vi "VP_RT_multiscan.vi"() -> ()   [LabVIEW 2015]
uses:
  Local or Remote.ctl
  State Enum.ctl
  Command Enum.ctl
  Controller Type.ctl
  Scan type.ctl
  EPICS Command Control.ctl
  <vilib>/Platform/TimedLoop/XDataNode/timing_clust.ctl
  <vilib>/Platform/TimedLoop/XDataNode/nitl_modes.ctl
  <vilib>/Platform/TimedLoop/XDataNode/wakeup.ctl
  Data Write Control.ctl
  <vilib>/FPGAPlugInAG/cRIO-9039/niLvFpga_Open_cRIO-9039.vi
  <vilib>/rvi/interface/common/dynamic/niFpgaDynamicAddResources.vi
  <vilib>/Utility/error.llb/Error Cluster From Error Code.vi
  <vilib>/rvi/errors/niLvFpgaAdjustHostInterfaceError.vi
  <vilib>/rvi/interface/common/niFpgaWaitOnOcc.vi
  <vilib>/FPGAPlugInAG/Dynamic/niLvFpga_Reset_Dynamic.vi
  <vilib>/FPGAPlugInAG/Dynamic/niLvFpga_Abort_Dynamic.vi
  <vilib>/FPGAPlugInAG/Dynamic/niLvFpga_Close_Dynamic.vi
  <vilib>/Platform/TimedLoop/XDataNode/XDataNode.xnode
  <vilib>/rvi/interface/nirviOpenFPGA/nirviOpenFPGA.xnode
  FPGA Bitfiles/VP_NanoPositioner_FPGA_Diagonal.lvbitx
  <vilib>/rvi/interface/nirviReadWriteControl/nirviReadWriteControl.xnode
  <vilib>/rvi/interface/nirviMethod/nirviMethod.xnode
  <vilib>/rvi/interface/nirviCloseFPGA/nirviCloseFPGA.xnode
  <vilib>/Platform/TimedLoop/XDataNode/XDNodeRunTimeDep.lvlib
  <vilib>/rvi/errors/niLvFpgaMergeErrorWithErrorCode.vi
  NiFpgaLv.dll
  <vilib>/rvi/interface/Simulation/niFpgaSimulationCallBeginRW.vi
  <vilib>/rvi/Analysis/host/Public/NI_FpgaMspHost.lvlib
  <vilib>/FPGAPlugInAG/Dynamic/niLvFpga_StopFifo_Dynamic.vi
  <vilib>/FPGAPlugInAG/Dynamic/niLvFpga_ReadFifo_Dynamic.vi
  <vilib>/NI_Real-Time Target Support.lvlib
  <vilib>/FPGAPlugInAG/Dynamic/niLvFpga_ConfigureFifo_Dynamic.vi
panel:
  in  "Tab Control":T1(tab)
  in  "Scan type":T2
  in  "Controller Type":T3
  out "Fly Scan Complete":bool
  out "XY actual":cluster{"Array":dbl[], "Array":dbl[]}(graph)
  out "XY Ref":cluster{"Array":dbl[], "Array":dbl[]}(graph)
  out "Elements Available in FIFO":u32(graph)
  out "Elements Remaining in FIFO":u32(graph)
  out "Reference and Actual positions":cluster{"t0":dbl, dbl, dbl[][]}(graph)
  in  "Timeout FPGA FIFO1":i32=40000000
  out "FIFO Timed Out":bool
  out "stop case":bool
  in  "Datalog Cases":T4(ring)=enum."Data Log 16"
  out "FIFO Timed Out?":bool
  out "Number of Elements":u32=1250
  out "Data Read Rate (Hz)":dbl=25000.000000000004
  out "Elements Remaining":u32
  in  "FIFO Timeout (ms)":i32=10000
  out "Actual Depth":u32=131068416
  in  "Requested Depth":u32=131068000
  out "2iddVELO:VP:X_End_nm":dbl=2000.0
  out "2iddVELO:VP:X_Start_nm":dbl=-2000.0
  out "EPICS Execute Command":bool
  out "2iddVELO:VP:Y_Start_nm":dbl=2000.0
  out "2iddVELO:VP:Y_End_nm":dbl=-2000.0
  out "2iddVELO:VP:Y_Step_Size_nm":dbl=50.0
  out "2iddVELO:VP:X_Step_Size_nm":dbl=50.0
  out "2iddVELO:VP:Trigger_Freq_Hz":dbl=1000.0
  out "2iddVELO:VP:Trig_DutyCycle_Per":dbl=99.0
  out "Iteration Duration RT Timed-Loop":i64=128
  in  "X Ramp Start (nm)":fxp<+/-,16,16>=-500.0
  in  "X Ramp End (nm)":fxp<+/-,16,16>=500.0
  in  "X Start Marker (nm)":fxp<+/-,58,25>
  in  "Y Ramp Start (nm)":fxp<+/-,16,16>=500.0
  in  "Y Ramp End (nm)":fxp<+/-,16,16>=-500.0
  in  "Y Step Size (nm)":fxp<+/-,16,16>=50.0
  in  "Y Start Marker (nm)":fxp<+/-,58,25>
  out "Fly Scan Running":bool
  out "Continue Run":bool
  out "X Ramp Period (usec)":fxp<+,24,24>=60000.0
  out "Y Ramp Period (usec)":fxp<+,24,24>=60000.0
  out "# of Hor Lines":fxp<+/-,34,18>=181.0 format="%.22g"
  in  "X Step Size (nm)":fxp<+/-,16,16>=50.0
  out "# of Points per Line":fxp<+/-,33,17>=180.0
  out "# Total Trigger Points":fxp<+/-,64,34>=32580.0
  out "sec per line":dbl=0.06
  out "line per sec (Hz)":dbl=16.666666666666668
  out "X Ramp Period DBL (usec)":dbl=60000.0 format="%#_6f"
  out "Total Scan Time (sec)":dbl=10.86
  in  "Controller Time Period (uSec)":u32=40
  in  "Controller Output Time Period (uSec)":u32=40
  in  "X Reference Time Period (uSec)":u32=40
  in  "Plant Output Time Period (uSec)":u32=40
  in  "Stop System (Careful!!)":bool
  in  "Datalog Time Period (uSec)":u32=40
  in  "Analog Input Time Period (uSec)":u32=40
  in  "Detector Trigger Time Period (uSec)":u32=40
  in  "Trigger Generation Time Period (uSec)":u32=40
  in  "Y Reference Time Period (uSec)":u32=40
  in  "Z Reference Time Period (uSec)":u32=40
  in  "Data Trigger Time Period (uSec)":u32=40
  in  "Reset All":bool
  in  "System Loop Type":enum16{"Open Loop", "Closed Loop"}(ring)
  in  "Base name":string="base_name"
  out "Trigger for Data":fxp<+/-,58,25>=1.0
  out "Data":fxp<+/-,58,25>[](array[numeric])
  out "Number of Data Strings":i32=5
  out "Mod6/DIO3":bool
  out "Mod5/DIO3":bool
  out "Mod4/DIO3":bool
  in  "Sample Z Stage Resolution (nm)":fxp<+,33,3>=0.5
  in  "Sample Y Stage Resolution (nm)":fxp<+,33,3>=0.5
  in  "Sample X Stage Resolution (nm)":fxp<+,33,3>=0.5
  in  "Optics Z Stage Resolution (nm)":fxp<+,33,3>=0.5
  in  "Optics Y Stage Resolution (nm)":fxp<+,33,3>=0.5
  in  "Optics X Stage Resolution (nm)":fxp<+,33,3>=0.5
  in  "Sample Z Reset":bool
  in  "Sample Y Reset":bool
  in  "Sample X Reset":bool
  out "Mod6/DIO2":bool
  out "Mod6/DIO1":bool
  out "Mod6/DIO0":bool=TRUE
  out "Mod5/DIO2":bool
  out "Mod5/DIO1":bool=TRUE
  out "Mod5/DIO0":bool
  out "Mod4/DIO2":bool=TRUE
  out "Mod4/DIO1":bool
  out "Mod4/DIO0":bool=TRUE
  in  "Optics Z Reset":bool
  in  "Optics Y Reset":bool
  in  "Optics X Reset":bool
  in  "Detector Trigger Lower Limit (V)":fxp<+/-,20,5>
  in  "Detector Trigger Upper Limit (V)":fxp<+/-,20,5>=5.0
  out "Detector Trigger (V)":fxp<+/-,20,5>
  out "Detector Trigger In Range?":bool=TRUE
  in  "Trigger High Period (usec)":fxp<+/-,64,45>=1250.0
  in  "Trigger Low Period (usec)":fxp<+/-,64,45>=1250.0
  in  "Trigger High Level (V)":fxp<+/-,20,5>=5.0
  in  "Trigger Low Level (V)":fxp<+/-,20,5>
  in  "Trigger Wave Generator":T5(ring)=enum."Square Wave 1"
  in  "DT Reference Amplitude (V)":fxp<+/-,40,17>=5.0
  in  "DT Reference DC Offset (V)":fxp<+/-,16,16>
  out "DT Frequency (periods/tick)":fxp<+,32,0>=7.500010542571545e-05
  out "DT Phase Offset (periods)":fxp<+,32,0>
  in  "DT Reset":bool
  out "DT Duty Cycle (periods)":fxp<+,32,0>=0.8799999998882413
  in  "DT phase offset (deg)":dbl format="%#.6g"
  in  "DT Frequency (Hz)":dbl=200.0 format="%#_6p"
  in  "DT duty cycle (%)":dbl=88.0 min=0.0 max=100.0 step=1.0
  in  "Z White Noise Seed":u32=4
  in  "Z White Noise Amplitude":u16=32767
  in  "Y White Noise Seed":u32=4
  in  "Y White Noise Amplitude":u16=32767
  in  "Z Reference Reset":bool
  in  "Y Reference Reset":bool
  in  "X Reference Reset":bool
  in  "Z Reference Wave Selection":T6(ring)=enum."Sine Wave"
  in  "X Reference Wave Selection":T7(ring)=enum."Custom Up Down Ramp"
  in  "Y Reference Wave Selection":T8(ring)=enum."Custom Ramp Wave"
  out "Z phase offset (periods)":fxp<+,32,0>
  out "Z frequency (periods/tick)":fxp<+,32,0>=1.25030055642128e-07 format="%.32g"
  in  "Z phase offset (deg)":dbl format="%#.6g"
  in  "Z frequency (Hz)":dbl=5.0 format="%#_6p"
  out "Y phase offset (periods)":fxp<+,32,0>
  out "Y frequency (periods/tick)":fxp<+,32,0>=5.005858838558197e-08 format="%.32g"
  in  "Y phase offset (deg)":dbl format="%#.6g"
  in  "Y frequency (Hz)":dbl=2.0 format="%#_6p"
  out "Z Stage Reference (nm)":fxp<+/-,58,25>
  out "Y Stage Reference (nm)":fxp<+/-,58,25>
  out "X Stage Reference (nm)":fxp<+/-,58,25>
  in  "X White Noise Seed":u32=4
  in  "X White Noise Amplitude":u16=32767
  in  "Z Reference DC Offset (nm)":fxp<+/-,15,15>
  in  "Y Reference DC Offset (nm)":fxp<+/-,16,16>
  in  "X Reference DC Offset (nm)":fxp<+/-,16,16>
  in  "Z Reference Amplitude (nm)":fxp<+/-,40,17>
  in  "Y Reference Amplitude (nm)":fxp<+/-,40,17>=100.0
  in  "X Reference Amplitude (nm)":fxp<+/-,40,17>=100.0
  out "X phase offset (periods)":fxp<+,32,0>
  out "X frequency (periods/tick)":fxp<+,32,0>=1.25030055642128e-07 format="%.32g"
  in  "X phase offset (deg)":dbl format="%#.6g"
  in  "X frequency (Hz)":dbl=5.0 format="%#_6p"
  in  "Scaling mV to V":fxp<+,33,10>=0.001000046730041504
  out "Heartbeat":bool=TRUE
  in  "System command":T9
  in  "Execute":bool
  out "Last Command Executed":T9
  in  "Optics and or Sample Stage":T10(ring)
  out "Remote Mode":bool
  in  "Local_Lock":bool
  out "Local or EPICS":T11
  out "Output filename":string
  out "Output path":path
  out "FPGA state":T12(ring)
  in  "cRIO data dir":string="/home/lvuser/natinst/data"
  out "RT Main Loop State":T13
  out "cRIO path":path
  out "Trigger Frequency (Hz)":dbl
  out "Trigger Duty Cycle (%)":dbl
  out "EPICS Scan Type":T2
  out "EPICS Controller Type":T3
  out "EPICS cRIO Command":T14
  out "Scan loop dt":i64
  in  "FIFO Timeout ratio":dbl=0.05
  in  "Z-Stage Scaling Direction":fxp<+/-,3,3>=-1.0
  in  "Y-Stage Scaling Direction":fxp<+/-,3,3>=-1.0
  in  "Mod 3 AI2 V to nm Scaling":fxp<+,47,18>=1000.0
  in  "Mod 3 AI1 V to nm Scaling":fxp<+,47,18>=1000.0
  in  "Mod 3 AI0 V to nm Scaling":fxp<+,47,18>=1000.0
  out "PI Z-Stage Input (V)":fxp<+/-,20,5>=-0.000732421875
  out "PI Y-Stage Input (V)":fxp<+/-,20,5>=0.005584716796875
  out "PI X-Stage Input (V)":fxp<+/-,20,5>=-0.00311279296875
  in  "Z-Stage nm to V Scaling":fxp<+/-,32,12>=0.0005397796630859375
  in  "Y-Stage nm to V Scaling":fxp<+/-,32,12>=0.0014200210571289062
  in  "X-Stage Scaling Direction":fxp<+/-,3,3>=-1.0
  in  "X-Stage nm to V Scaling":fxp<+/-,32,12>=0.0005359649658203125
  in  "Controller Output Lower Limit":fxp<+/-,20,5>=-5.0
  in  "Controller Output Upper Limit":fxp<+/-,20,5>=5.0
  in  "FPGA Wait Timer (ms)":u16=50
  in  "Pre-Scan pause (ms)":u32=250
  in  "Readback Loop time between iterations (ms)":u32=10
  out "Measured Datalog Time Period (Ticks)":u32=1600
  out "Measured Datalog Loop Rate (secs)":dbl=3.9999999999999996e-05
  out "Measured Datalog Loop Rate (kHz)":dbl=25.000000000000004
  out "Measured Counter Loop Rate (secs)":dbl
  out "Measured Counter Loop Rate (MHz)":dbl=inf
  out "Measured X Reference Loop Rate (secs)":dbl=3.9999999999999996e-05
  out "Measured X Reference Loop Rate (kHz)":dbl=25.000000000000004
  out "Measured X Reference Time Period (Ticks)":u32=1600
  out "Measured Controller Loop Rate (kHz)":dbl=25.000000000000004
  out "Measured Controller Output Loop Rate (secs)":dbl=3.9999999999999996e-05
  out "Measured Controller Output Loop Rate (kHz)":dbl=25.000000000000004
  out "Measured Plant Output Loop Rate (secs)":dbl=3.9999999999999996e-05
  out "Measured Plant Output Loop Rate (kHz)":dbl=25.000000000000004
  out "Measured Controller Loop Rate (secs)":dbl=3.9999999999999996e-05
  out "Measured Controller Time Period (Ticks)":u32=1600
  out "Data Read Period (sec)":dbl=3.9999999999999996e-05
  out "Measured Controller Output Time Period (Ticks)":u32=1600
  out "Measured Plant Output Time Period (Ticks)":u32=1600
  out "Measured Counter Time Period (Ticks)":u32
  out "32 bit Count Optics X":i32
  out "32 bit Count Optics  Y":i32
  out "32 bit Count Optics  Z":i32
  out "32 bit Count Sample X":i32
  out "32 bit Count Sample  Y":i32=2
  out "32 bit Count Sample  Z":i32=-4
  out "Optics X Stage Displacement (nm)":fxp<+/-,58,25>=-1.0
  out "Optics Y Stage Displacement (nm)":fxp<+/-,58,25>
  out "Optics Z Stage Displacement (nm)":fxp<+/-,58,25>
  out "Sample X Stage Displacement (nm)":fxp<+/-,58,25>=-0.5
  out "Sample Y Stage Displacement (nm)":fxp<+/-,58,25>=1.5
  out "Sample Z Stage Displacement (nm)":fxp<+/-,58,25>=-1.0
  out "Measured Analog Input Time Period (Ticks)":u32=1600
  out "Measured Analog Input Loop Rate (secs)":dbl=3.9999999999999996e-05
  out "Measured Analog Input Loop Rate (kHz)":dbl=25.000000000000004
  out "Measured Detector Trigger Time Period (Ticks)":u32=1600
  out "Measured Trigger Gen Time Period (Ticks)":u32=1600
  out "Measured Y Reference Time Period (Ticks)":u32=1600
  out "Measured Z Reference Time Period (Ticks)":u32=1600
  out "Measured Y Reference Loop Rate (secs)":dbl=3.9999999999999996e-05
  out "Measured Y Reference Loop Rate (kHz)":dbl=25.000000000000004
  out "Measured Z Reference Loop Rate (secs)":dbl=3.9999999999999996e-05
  out "Measured Z Reference Loop Rate (kHz)":dbl=25.000000000000004
  out "Measured Data Trigger Time Period (Ticks)":u32=1600
  out "X-Stage Input In Range?":bool=TRUE
  out "Y-Stage Input In Range?":bool=TRUE
  out "Z-Stage Input In Range?":bool=TRUE
  in  "file path soscoeff_xx1 Hinf":path=path "/home/lvuser/natinst/controllers/Kxx_1_Gxx_matched_dow_16ord_mVpnm_cd8a3_AvTio9_X5nm_500pm_all_40us_soscof_xx1.mat"
  in  "file path sos gain SF Controller_xx1 Hinf":path=path "/home/lvuser/natinst/controllers/Kxx_1_Gxx_matched_dow_16ord_mVpnm_cd8a3_AvTio9_X5nm_500pm_all_40us_soscof_xx2.mat"
  in  "file path soscoeff_yy1 Hinf":path=path "/home/lvuser/natinst/controllers/Kyy_trial_1_Gyy_matched_dow_8ord_mVpnm_cd8a3_AvTio9_Y5nm_500pm_all_40us_soscof_yy1.mat"
  in  "file path sos gain SF Controller_yy1 Hinf":path=path "/home/lvuser/natinst/controllers/Kyy_trial_1_Gyy_matched_dow_8ord_mVpnm_cd8a3_AvTio9_Y5nm_500pm_all_40us_soscof_yy2.mat"
  in  "file path soscoeff_zz1 Hinf":path=path "/home/lvuser/natinst/controllers/Kzz_1_Gzz_matched_dow_29ord_mVpnm_cd8a3_AvTio9_Z5nm_500pm_all_40us_soscof_zz1.mat"
  in  "file path sos gain SF Controller_zz1 Hinf":path=path "/home/lvuser/natinst/controllers/Kzz_1_Gzz_matched_dow_29ord_mVpnm_cd8a3_AvTio9_Z5nm_500pm_all_40us_soscof_zz2.mat"
  in  "file path soscoeff_xx1 PID":path=path "/home/lvuser/natinst/controllers/Kxx_pid_2_Gxx_tustin_2ord_mVpnm_cd8a3_soscof_xx1.mat"
  in  "file path sos gain SF Controller_xx1 PID":path=path "/home/lvuser/natinst/controllers/Kxx_pid_2_Gxx_tustin_2ord_mVpnm_cd8a3_soscof_xx2.mat"
  in  "file path soscoeff_yy1 PID":path=path "/home/lvuser/natinst/controllers/Kyy_pid_4_Gyy_tustin_2ord_mVpnm_cd8a3_soscof_yy1.mat"
  in  "file path sos gain SF Controller_yy1 PID":path=path "/home/lvuser/natinst/controllers/Kyy_pid_4_Gyy_tustin_2ord_mVpnm_cd8a3_soscof_yy2.mat"
  in  "file path soscoeff_zz1 PID":path=path "/home/lvuser/natinst/controllers/Kzz_pid_2_Gzz_tustin_2ord_mVpnm_cd8a3_soscof_zz1.mat"
  in  "file path sos gain SF Controller_zz1 PID":path=path "/home/lvuser/natinst/controllers/Kzz_pid_2_Gzz_tustin_2ord_mVpnm_cd8a3_soscof_zz2.mat"
  out "-a01(2) xx1c":fxp<+/-,64,9>[](array[numeric])=[0.637785025840232, 0.9924182654286198, 1.8461027816316544, 0.8635404845716299, 1.0670555456779864, 1.6350703383821101, 1.6323955588345012, 1.1102241390539636, 0.0, 0.0, 0.0, 0.0, 0.0, 0.0, 0.0, 0.0, 0.0, 0.0, 0.0, 0.0]
  out "-a02(2) xx1c":fxp<+/-,64,9>[](array[numeric])=[-0.999855815746439, -0.9676991072632725, -0.9642268720534838, -0.9446498323360957, -0.9442808087139987, -0.7547983908829242, -0.6690016013017409, -0.11027986125857198, 0.0, 0.0, 0.0, 0.0, 0.0, 0.0, 0.0, 0.0, 0.0, 0.0, 0.0, 0.0]
  out "b01(2) xx1c":fxp<+/-,64,9>[](array[numeric])=[-0.6378105164532328, -1.0062332697665268, -1.8762916543815855, -0.8616288879491845, -1.0856571140792324, -1.6862585929720944, -1.743591709663851, -0.6129835805090948, 0.0, 0.0, 0.0, 0.0, 0.0, 0.0, 0.0, 0.0, 0.0, 0.0, 0.0, 0.0]
  out "b02(2) xx1c":fxp<+/-,64,9>[](array[numeric])=[0.9999102047610771, 0.9971375605901365, 0.9926840301018772, 0.9509648854364836, 0.9563369558920378, 0.7818900462139817, 0.7642575436257291, 3.0531133177191805e-16, 0.0, 0.0, 0.0, 0.0, 0.0, 0.0, 0.0, 0.0, 0.0, 0.0, 0.0, 0.0]
  out "sos gain SF Controller xx1c":fxp<+/-,42,9>=-0.1625035791657865
  out "-a01(2) yy1c":fxp<+/-,64,9>[](array[numeric])=[1.8740229377643998, 1.3096977339382483, 1.7453886241944765, 0.2668895009727739, 0.0, 0.0, 0.0, 0.0, 0.0, 0.0, 0.0, 0.0, 0.0, 0.0, 0.0, 0.0, 0.0, 0.0, 0.0, 0.0]
  out "-a02(2) yy1c":fxp<+/-,64,9>[](array[numeric])=[-0.9732703278433918, -0.5194903821190732, -0.7453924481836136, -2.7755575615628914e-17, 0.0, 0.0, 0.0, 0.0, 0.0, 0.0, 0.0, 0.0, 0.0, 0.0, 0.0, 0.0, 0.0, 0.0, 0.0, 0.0]
  out "b01(2) yy1c":fxp<+/-,64,9>[](array[numeric])=[-1.8979173162254057, -1.8463149313261074, -1.7151162246453355, -0.006444279582847878, 0.0, 0.0, 0.0, 0.0, 0.0, 0.0, 0.0, 0.0, 0.0, 0.0, 0.0, 0.0, 0.0, 0.0, 0.0, 0.0]
  out "b02(2) yy1c":fxp<+/-,64,9>[](array[numeric])=[0.9969084979865663, 0.9421233904433339, 0.7362048104846675, 0.0, 0.0, 0.0, 0.0, 0.0, 0.0, 0.0, 0.0, 0.0, 0.0, 0.0, 0.0, 0.0, 0.0, 0.0, 0.0, 0.0]
  out "sos gain SF Controller yy1c":fxp<+/-,42,9>=-1.480983349494636
  out "-a01(2) zz1c":fxp<+/-,64,9>[](array[numeric])=[0.6242394224317618, 1.8967038692417004, 0.6659160318030806, 1.7792660019034106, 1.6870099721477447, 0.6417945190222861, 1.4838029149808185, 1.8456549628851837, 1.2189509782386598, 0.9933314517253298, 1.0158915520299678, 0.8863484387433826, 0.026837806879254994, 1.8269783715122585, 0.22448441435364225, 0.0, 0.0, 0.0, 0.0, 0.0]
  out "-a02(2) zz1c":fxp<+/-,64,9>[](array[numeric])=[-0.9983298461163967, -0.9972287452752734, -0.995744457243837, -0.9947210838396919, -0.9925914602095722, -0.9920974045271405, -0.9881915357970101, -0.9800069383591395, -0.9760641145386646, -0.9508624135515895, -0.9242774595356998, -0.655945641403593, -0.008661844724279444, -0.8269827070369743, 0.0, 0.0, 0.0, 0.0, 0.0, 0.0]
  out "b01(2) zz1c":fxp<+/-,64,9>[](array[numeric])=[-0.6245671059510156, -1.897930093390194, -0.6670970070931089, -1.7670265604573054, -1.6833314913922348, -0.6327437892303018, -1.5025901530730128, -1.8636454269915796, -1.1210694827766767, -0.9982206064398196, -1.0326369335418408, -1.1342635673267367, -1.6852506306166828, -0.9843740162364313, -1.7208456881689926e-15, 0.0, 0.0, 0.0, 0.0, 0.0]
  out "b02(2) zz1c":fxp<+/-,64,9>[](array[numeric])=[0.9973135069419645, 0.9951302056171929, 0.9993435624612031, 0.9919371251860779, 0.994931751453586, 0.9881092761723503, 0.9884874399279107, 0.9977145546300196, 0.9725302934743221, 0.9855561672767964, 0.9893454712398023, 0.846212786518208, 0.7855598927779743, 0.0978075435519738, 0.0, 0.0, 0.0, 0.0, 0.0, 0.0]
  out "sos gain SF Controller zz1c":fxp<+/-,42,9>=-0.1988595259608701
  out "error out (Sig Gen)":errorcluster
  out "FPGA error monitor":errorcluster
  out "FPGA end run error":errorcluster
  out "Timed Loop (end error)":errorcluster
  out "error out (Sig Gen) 2":errorcluster
  out "error out (Sig Gen) 3":errorcluster
  out "error out (Sig Gen) 4":errorcluster
  out "Main Loop error":errorcluster
  out "Main Loop Iterations":i32
  out "RT error":errorcluster
  out "Command Loop Error":errorcluster
  out "Readback error":errorcluster
  out "FPGA wait error":errorcluster
  out "Coeff file import error":errorcluster
  out "Readback loop Iterations":i32
  out "Command Loop Iterations":i32
  out "Heartbeat Loop Iterations":i32
  out "EPICS command error":errorcluster
  out "Reduced Array of States":T13[](array[typedef])
  out "2iddVELO:VP:Scan_Type":string
  out "2iddVELO:VP:Controller_Type":string
  out "2iddVELO:VP:cRIO_Command":string
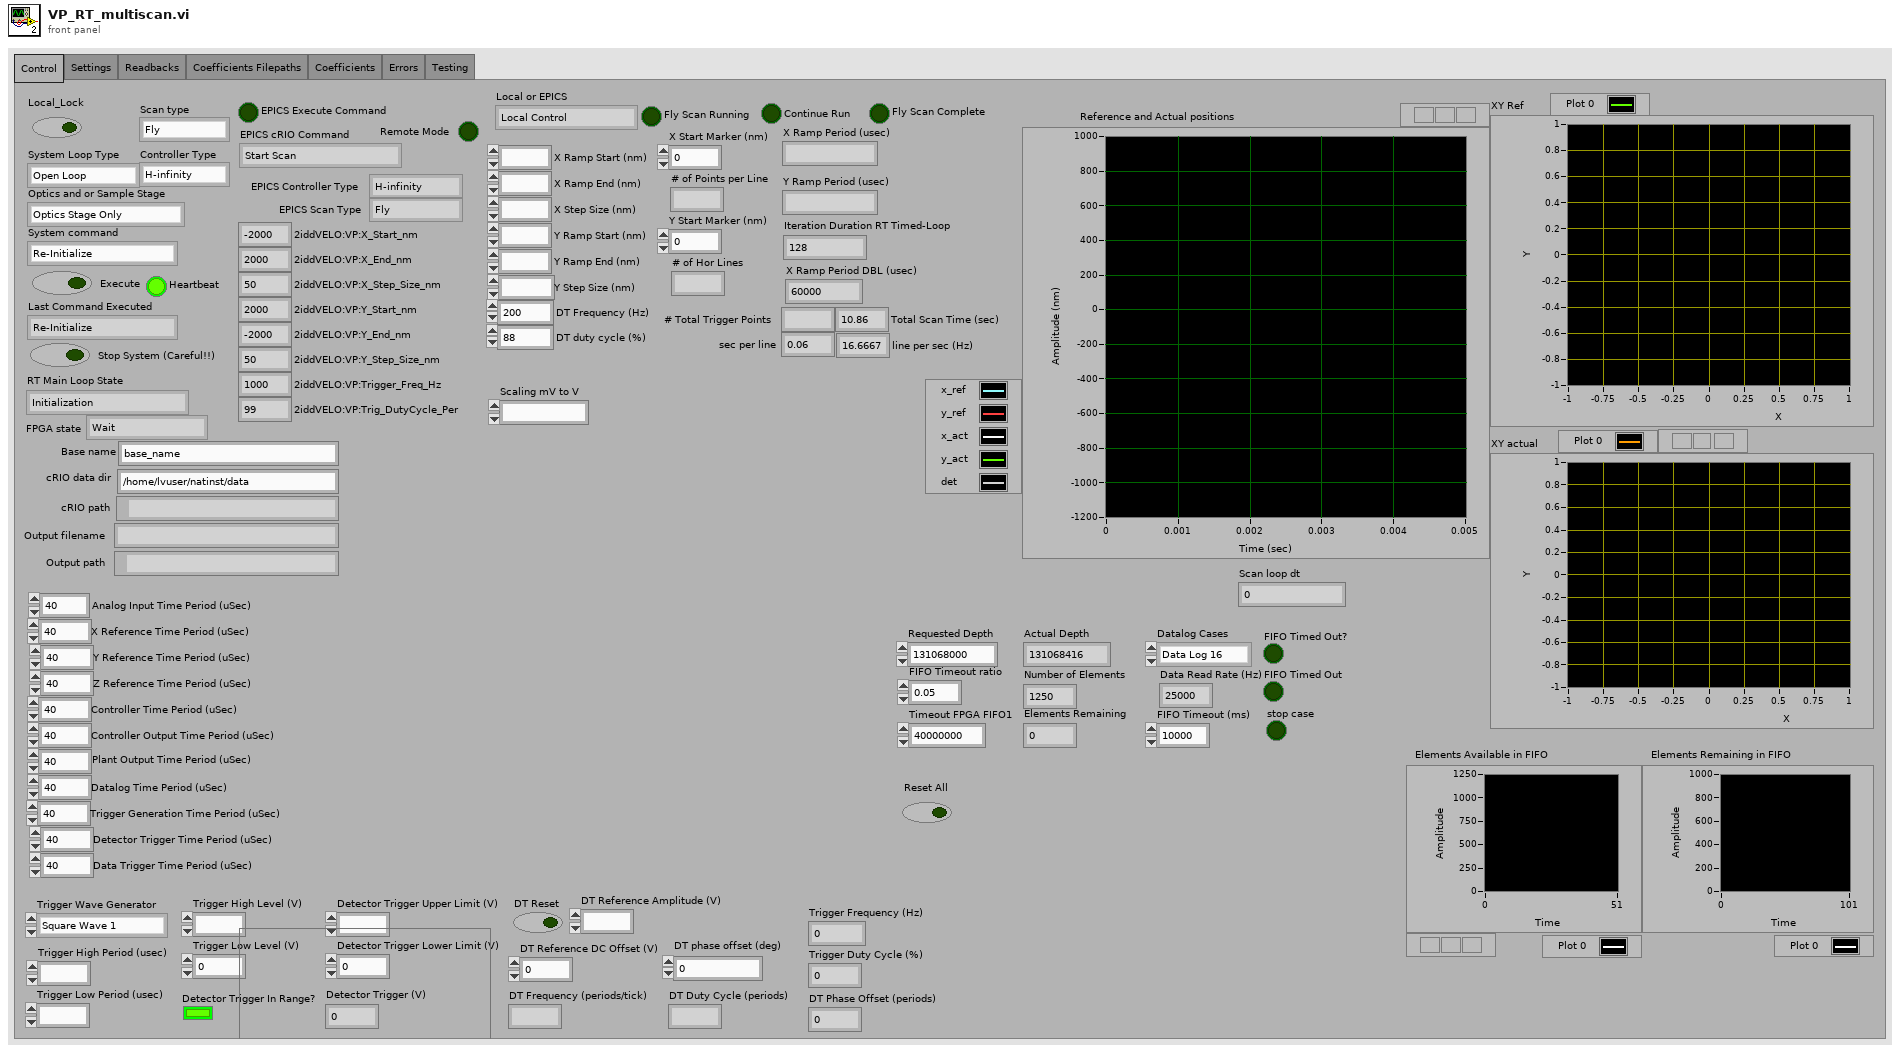
[diagram p1: front panel]
types:
  T1 = enum32{"Control", "Settings", "Readbacks", "Coefficients Filepaths", "Coefficients", "Errors", "Testing"}
  T2 = typedef "Scan type.ctl" = enum16{"Fly", "Step"}
  T3 = typedef "Controller Type.ctl" = enum16{"H-infinity", "PID"}
  T4 = enum16{"Data Log 1", "Data Log 2", "Data Log 3", "Data Log 4", "Data Log 5", "Data Log 6", "Data Log 7", "Data Log 8", "Data Log 9", "Data Log 10", "Data Log 11", "Data Log 12", "Data Log 13", "Data Log 14", "Data Log 15", "Data Log 16"}
  T5 = enum16{"Custom Square Wave ", "Square Wave 1", "Square Wave 2"}
  T6 = enum16{"Constant", "Sine Wave", "Sawtooth Wave", "Square Wave", "Filtered White Noise"}
  T7 = enum16{"Constant", "Sine Wave", "Custom Up Down Ramp", "Filtered White Noise"}
  T8 = enum16{"Constant", "Sine Wave", "Custom Ramp Wave", "Filtered White Noise"}
  T9 = typedef "Command Enum.ctl" = enum16{"Re-Initialize ", "Update Scan Settings", "Scan", "Stop Scan", "Restart FPGA", "Stop System"}
  T10 = enum16{"Optics Stage Only", "Optics and Sample Stage"}
  T11 = typedef "Local or Remote.ctl" = enum16{"Local Control", "EPICS Control"}
  T12 = enum16{"Wait", "Start Run", "Run", "End Run", "Shutdown"}
  T13 = typedef "State Enum.ctl" = enum16{"Initialization", "Import Controller coeffs", "Update Controller Info", "Wait", "Update Reference Info", "Update Detector Trigger Info", "Update Datalog Info", "Check FPGA Status", "Pre-Scan", "Start Scan", "Step Scanning", "Fly Scanning", "End Scan", "Restart FPGA", "Stop FPGA"}
  T14 = typedef "EPICS Command Control.ctl" = enum16{"Start Scan", "Stop Scan", "Reload Controller"}
  T15 = typedef "XDNodeRunTimeDep.lvlib/timing_clust.ctl" = cluster{"Expected End [f-1]":u64, "Actual End [f-1]":u64, "Finished Late? [f-1]":bool, "Expected End [i-1]":u64, "Actual End [i-1]":u64, "Finished Late? [i-1]":bool, "Expected Start [i]":u64, "Actual Start [i]":u64, "Expected Start [f]":u64, "Actual Start [f]":u64, "Source Name":string, "Structure Name":string, "Period":i64, "Deadline":i64, "Offset":i64, "Start":i64, "Priority":i32, "Timeout":i32, "Mode":T16, "Wakeup Reason":T17, "Error":errorcluster, "Source Type":string, "Secondary Source Type":string, "Global End Time":u64, "Global Start Time":u64, "Frame Duration":u64, "Iteration Duration":u64, "Assigned CPU":i32, "I/O Scan Engine Mode":u32}
  T16 = typedef "XDNodeRunTimeDep.lvlib/nitl_modes.ctl" = enum32{"No Change", "Process missed periods, maintain original phase", "Discard missed periods, maintain original phase", "Process missed periods, ignore original phase", "Discard missed periods, ignore original phase"}
  T17 = typedef "XDNodeRunTimeDep.lvlib/wakeup.ctl" = enum32{"Normal", "Aborted", "Asynchronous wakeup", "Timing source error", "Timed loop error", "Timeout"}
  T18 = typedef "Data Write Control.ctl" = enum16{"Initialize", "Read", "Write", "Close"}
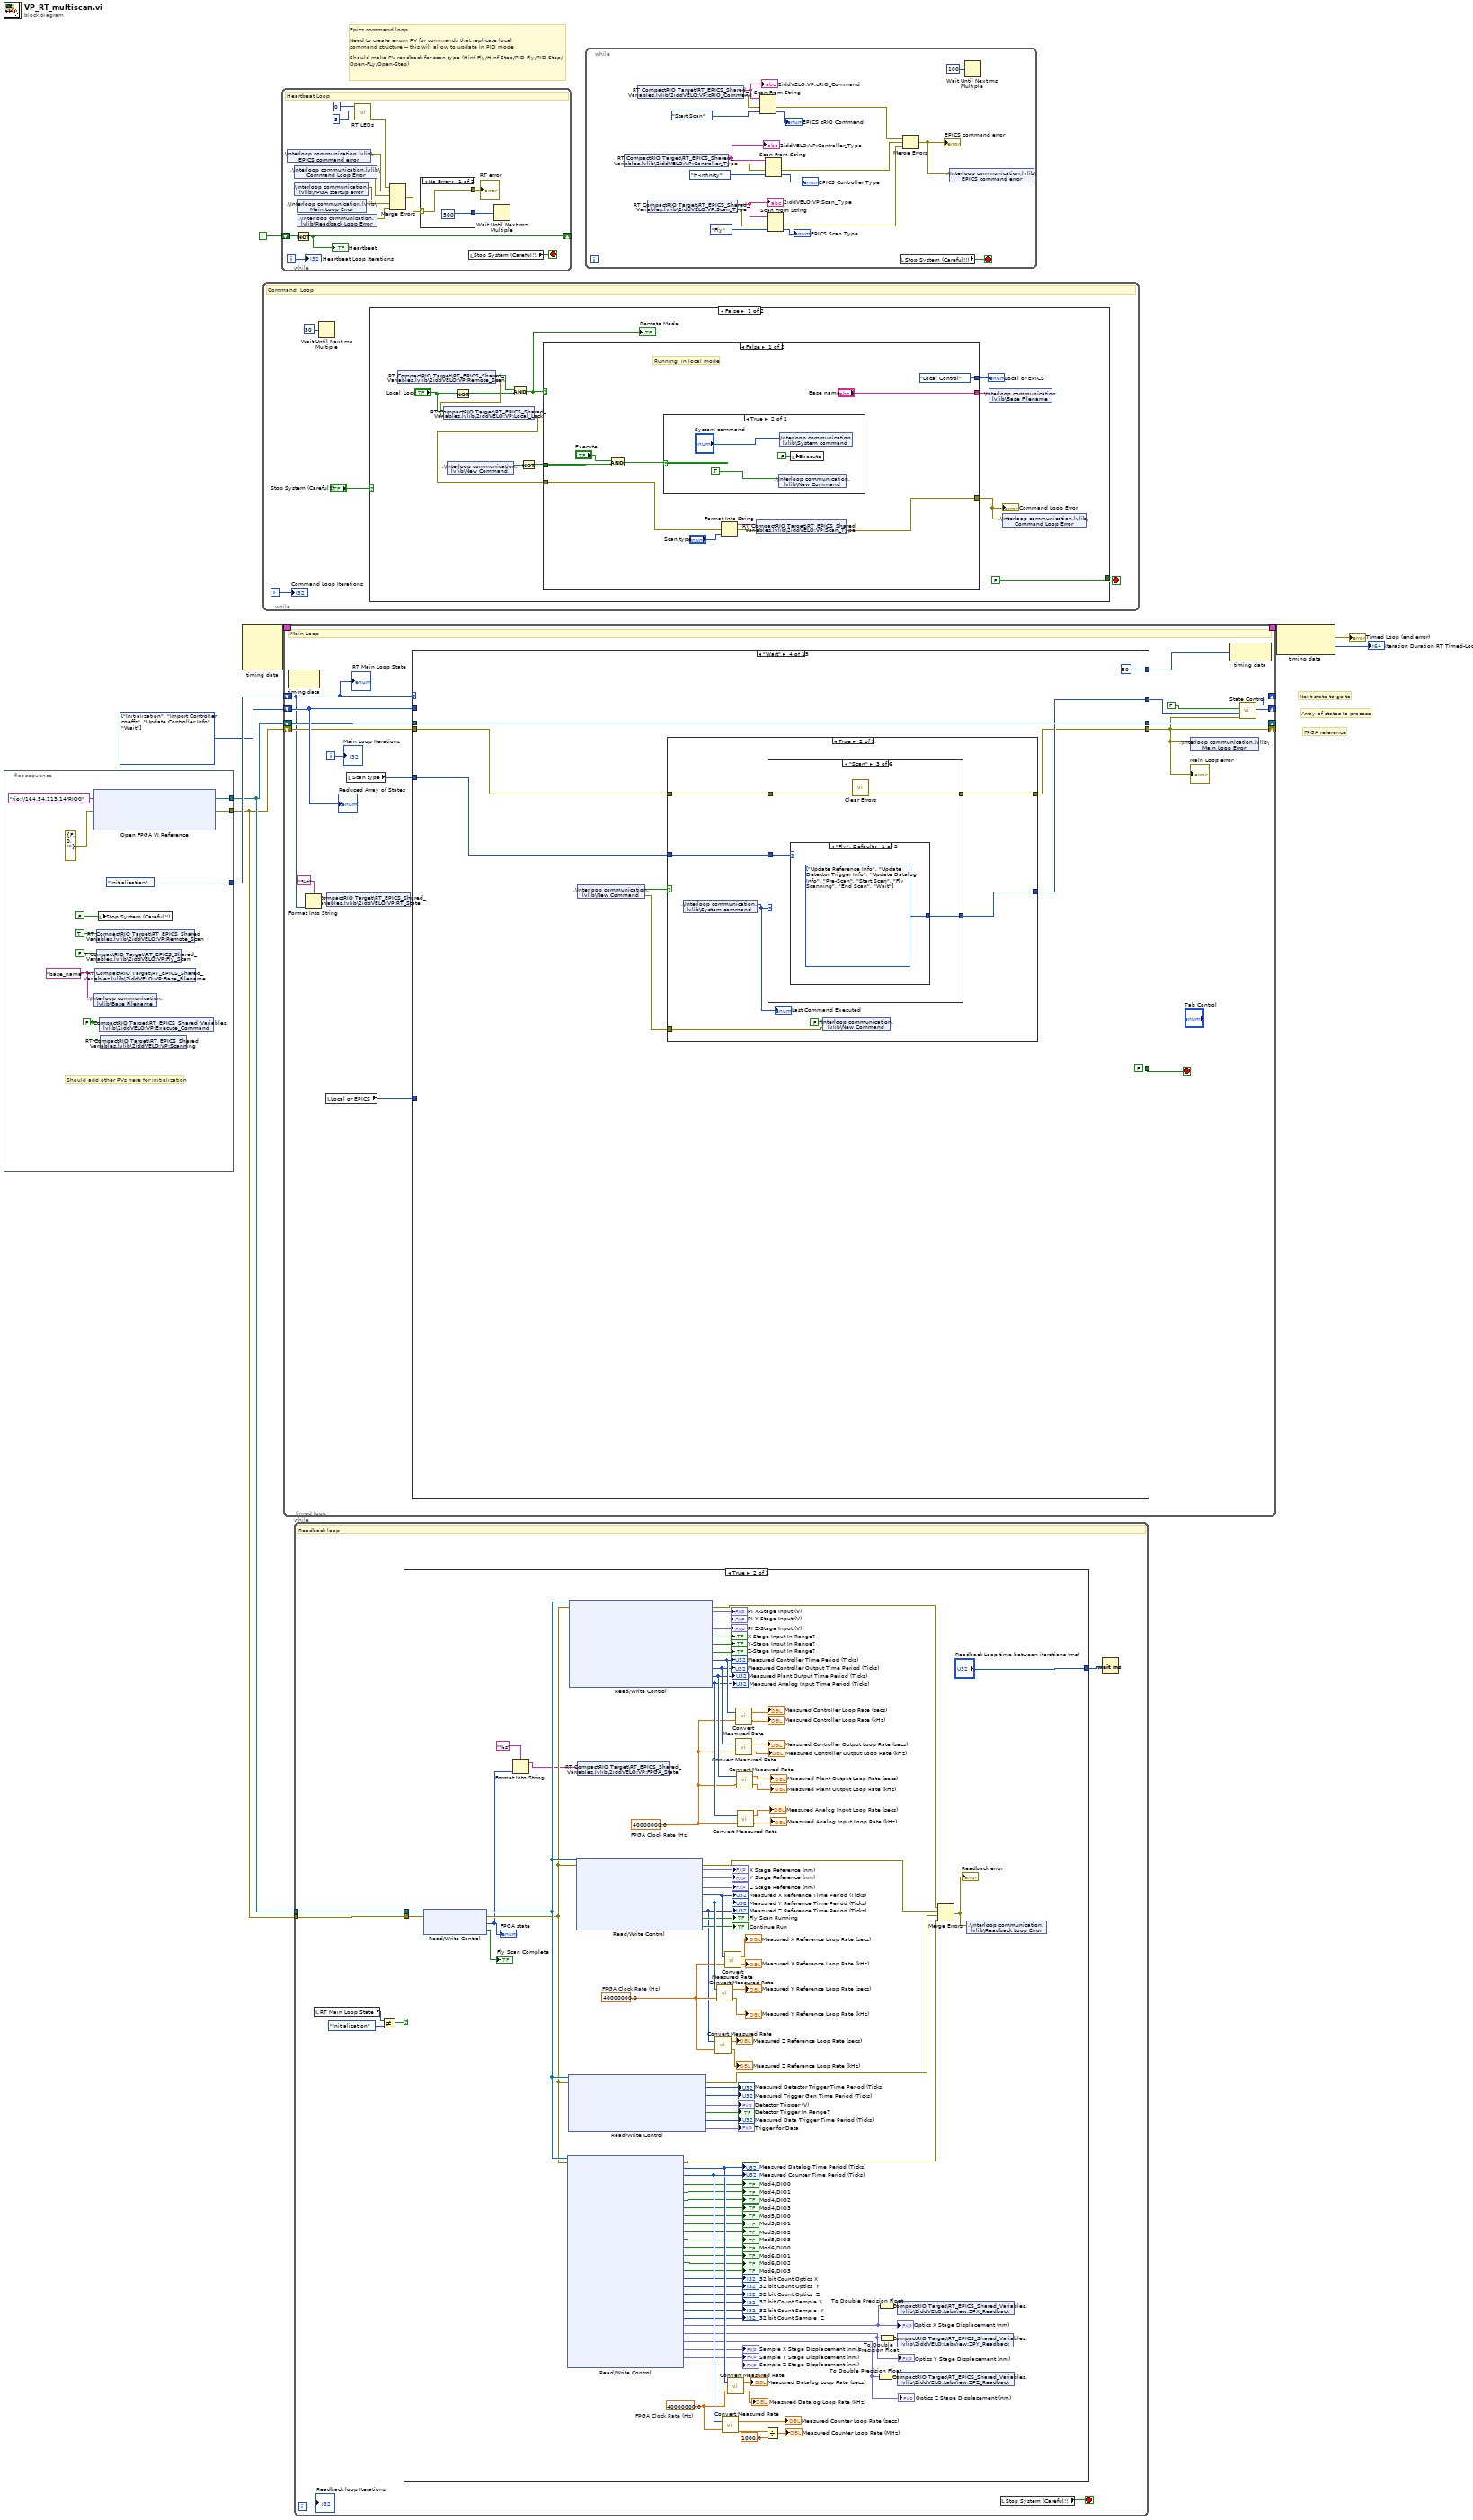
[diagram p0: block diagram]
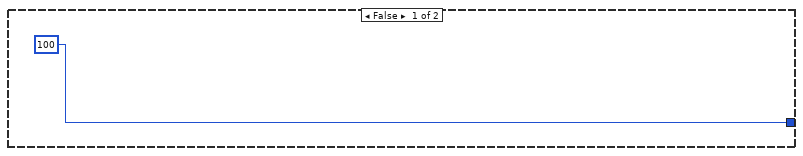
[diagram p2: hidden frame]
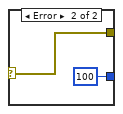
[diagram p3: hidden frame]
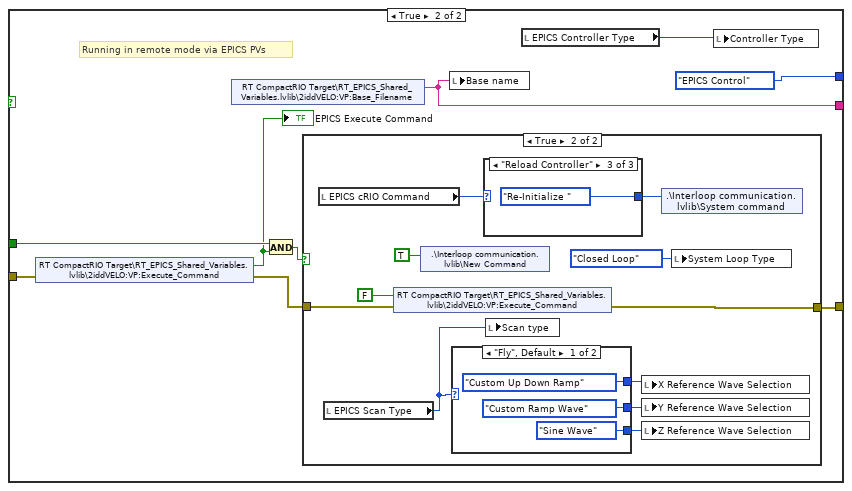
[diagram p5: hidden frame]
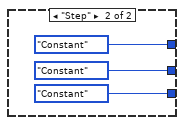
[diagram p7: hidden frame]
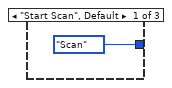
[diagram p8: hidden frame]
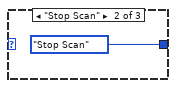
[diagram p9: hidden frame]
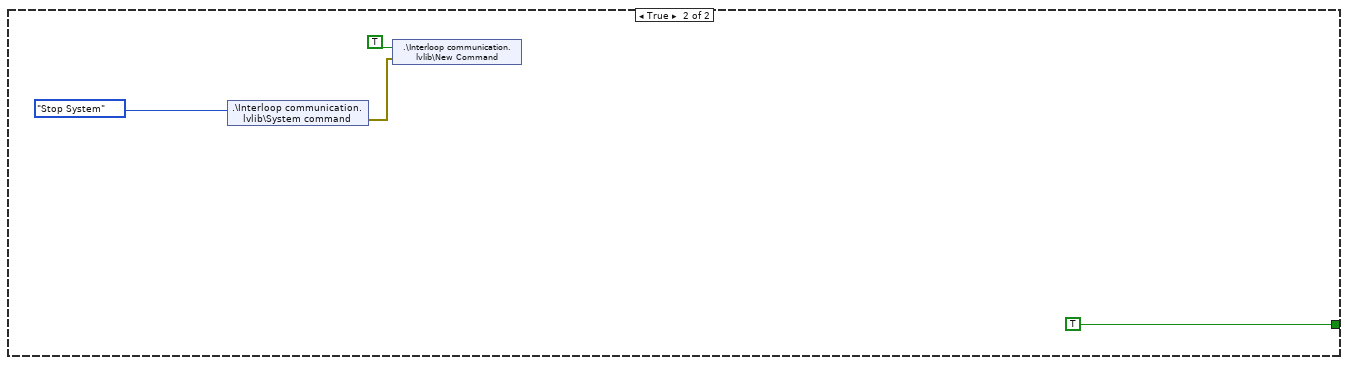
[diagram p10: hidden frame]
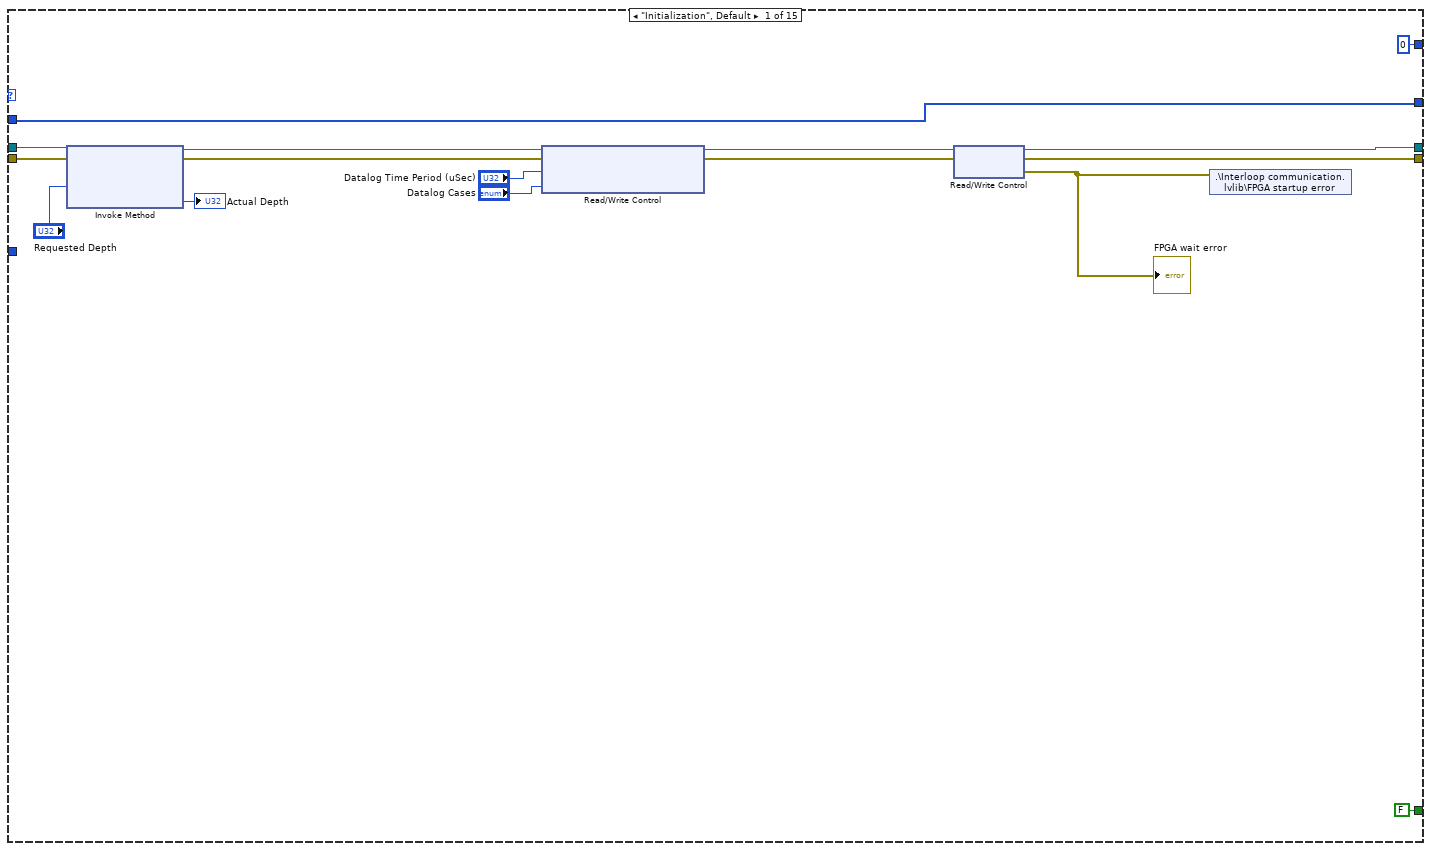
[diagram p11: hidden frame]
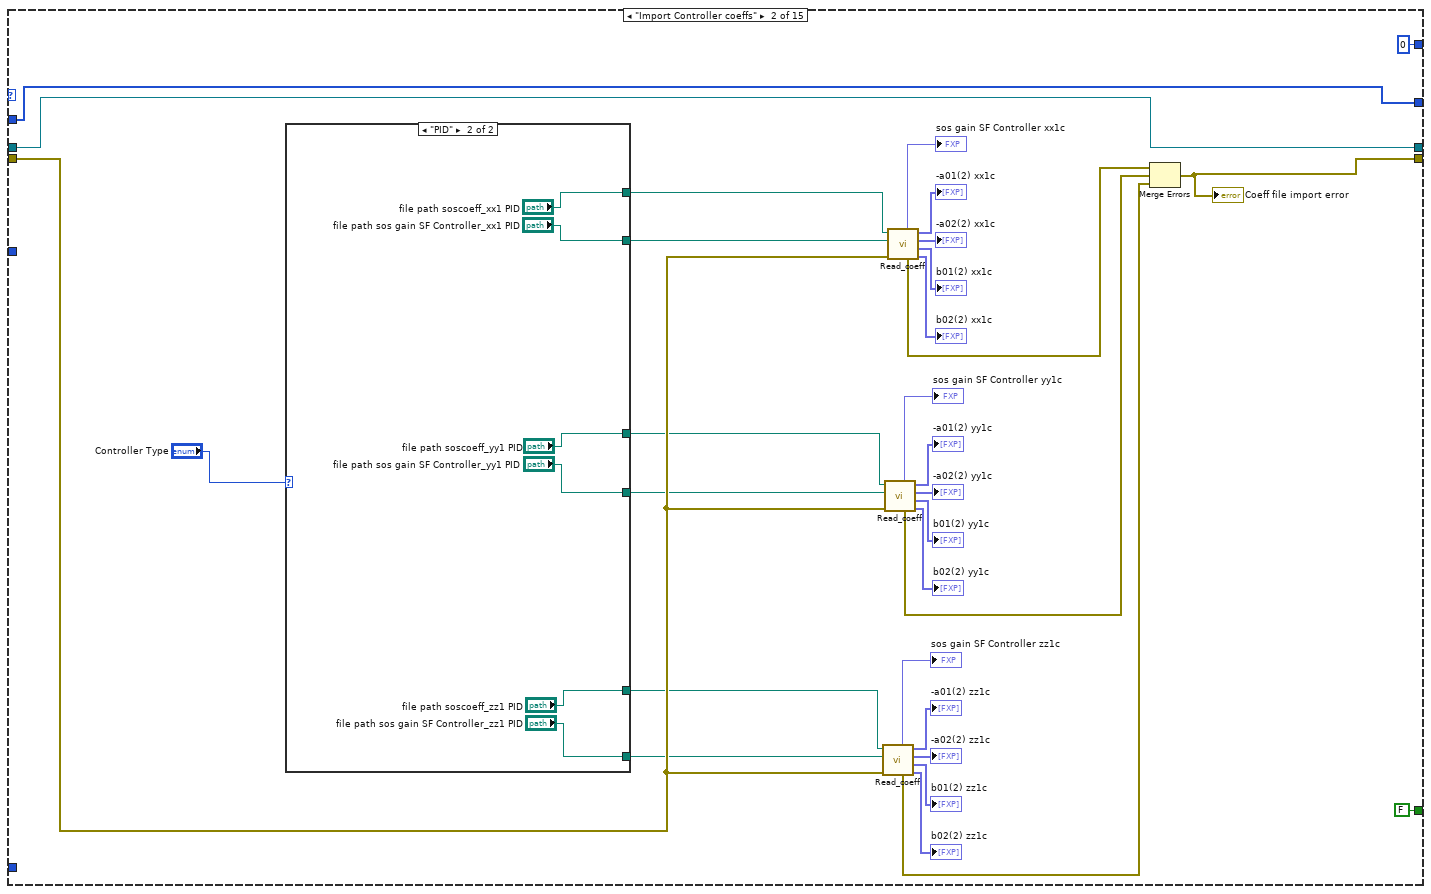
[diagram p12: hidden frame]
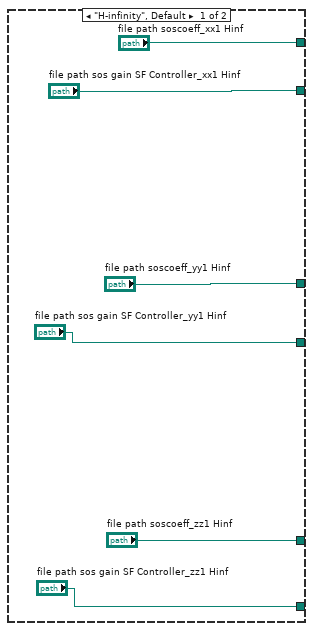
[diagram p13: hidden frame]
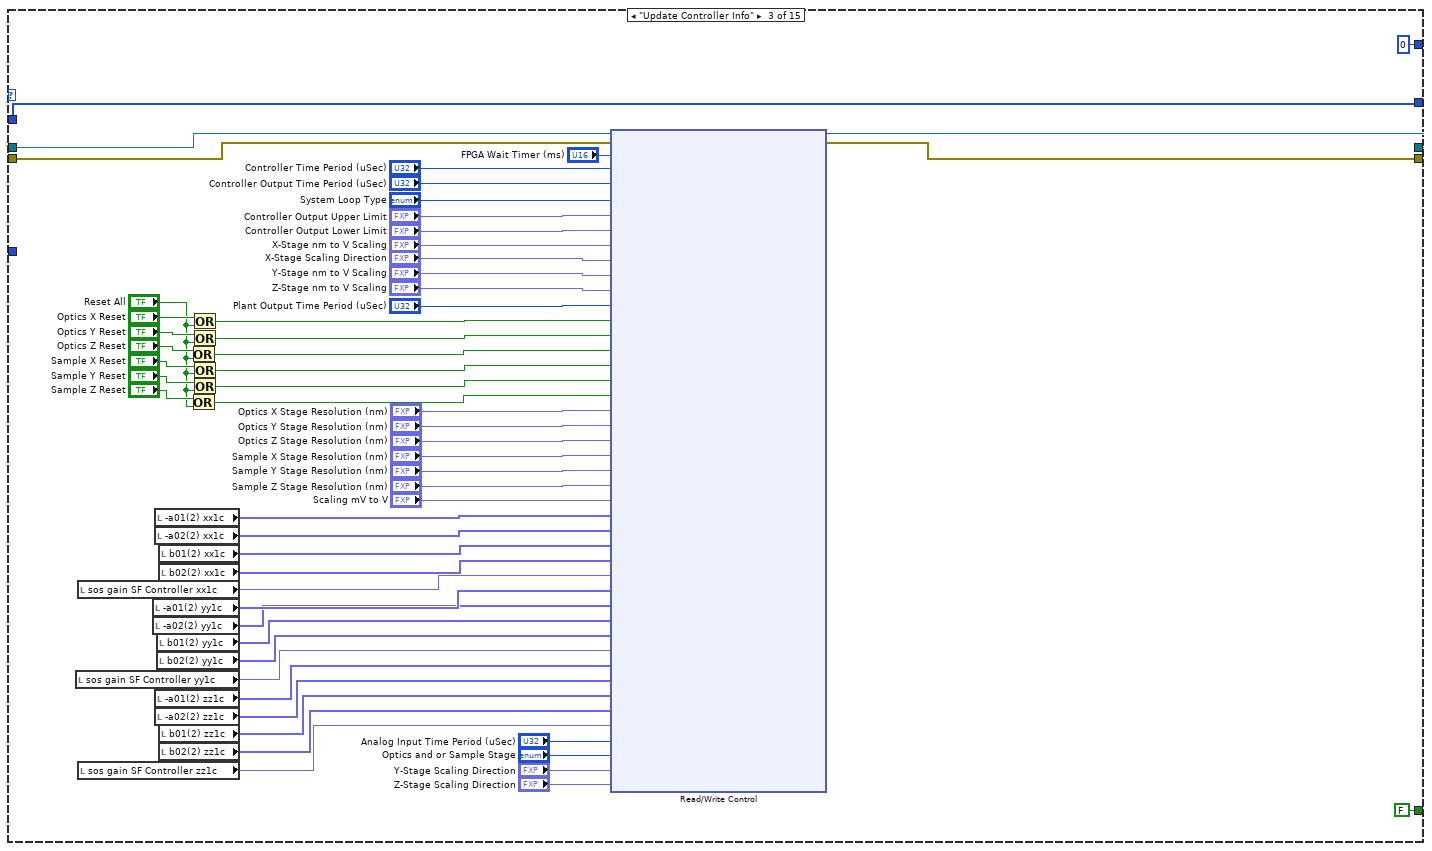
[diagram p14: hidden frame]
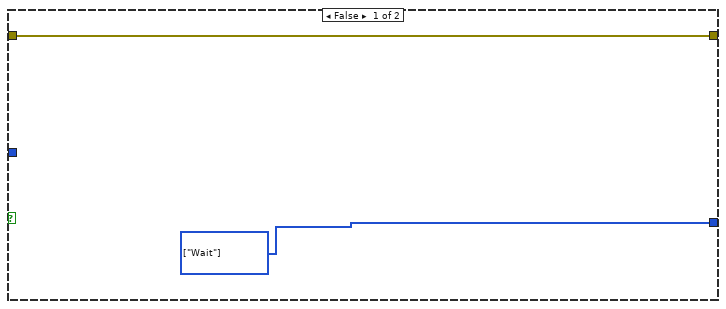
[diagram p15: hidden frame]
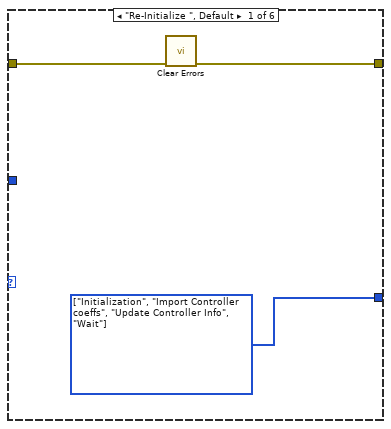
[diagram p16: hidden frame]
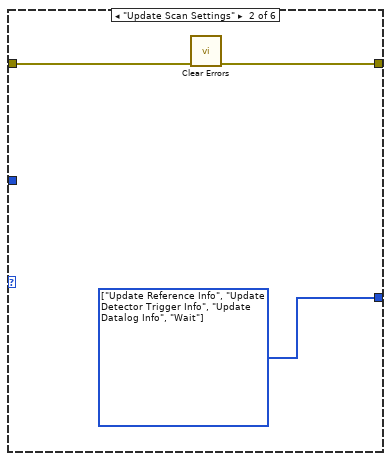
[diagram p17: hidden frame]
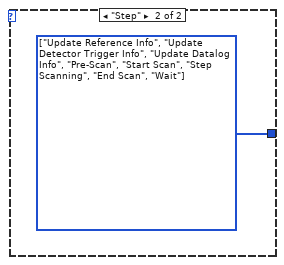
[diagram p18: hidden frame]
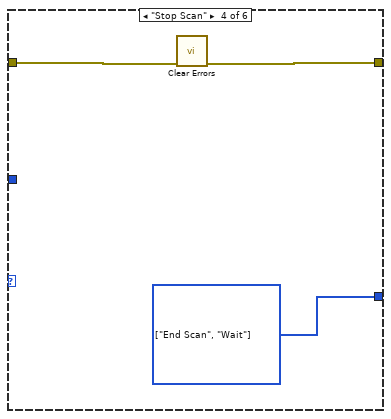
[diagram p19: hidden frame]
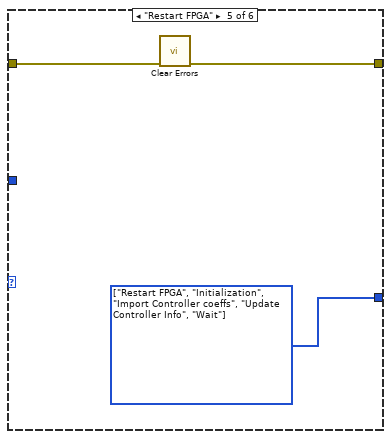
[diagram p20: hidden frame]
diagram:
  w3 = T13[] [enum."Initialization", enum."Import Controller coeffs", enum."Update Controller Info", enum."Wait"] items=["Initialization", "Import Controller coeffs", "Update Controller Info", "Wait", "Update Reference Info", "Update Detector Trigger Info", "Update Datalog Info", "Check FPGA Status", "Pre-Scan", "Start Scan", "Step Scanning", "Fly Scanning", "End Scan", "Restart FPGA", "Stop FPGA"] ("Reduced Array of States")
  # "Epics command loop\n\nNeed to create enum PV for commands that replicate local\ncommand structure -- this will allow to update in PID mode\n\nShould make PV readback for scan type (Hinf-Fly/Hinf-Step/PID-Fly/PID-Step/\nOpen-FLy/Open-Step)"
  # "FPGA reference"
  # "Array of states to process"
  # "Next state to go to"
  n1 = flat-sequence {
    tunnel: [State_Enum."Initialization" ("States")] -> w4
    tunnel: [w16] -> w1
    tunnel: [w15] -> w2
    frame #0 {
      w10 = FALSE ("Start_Scan")
      w13 = "base_name" ("Base_Filename")
      # "Should add other PVs here for initialization"
      n2 = xnode ("Open FPGA VI Reference")("error in"=errorcluster {"status"=FALSE, "code"=0, "source"=""} ("error constant"), "resource name"=tag "rio://164.54.113.14/RIO0") -> ("FPGA VI Reference Out"=w15:refnum<k20>, "error out"=w16:errorcluster)
      n3 = shared-variable ".\\Interloop communication.lvlib\\Base Filename"(w13) -> ()  [unwired: 1 in, 1 out]
      n4 = shared-variable "RT CompactRIO Target\\RT_EPICS_Shared_Variables.lvlib\\2iddVELO:VP:Base_Filename"(w13) -> ()  [unwired: 1 in, 1 out]
      n5 = shared-variable "RT CompactRIO Target\\RT_EPICS_Shared_Variables.lvlib\\2iddVELO:VP:Remote_Scan"(TRUE ("Remote_Scan")) -> ()  [unwired: 1 in, 1 out]
      n6 = shared-variable "RT CompactRIO Target\\RT_EPICS_Shared_Variables.lvlib\\2iddVELO:VP:Fly_Scan"(FALSE ("Fly_Scan")) -> ()  [unwired: 1 in, 1 out]
      n7 = local write "Stop System (Careful!!)"(FALSE ("Stop")) -> ()
      n8 = shared-variable "RT CompactRIO Target\\RT_EPICS_Shared_Variables.lvlib\\2iddVELO:VP:Execute_Command"(w10) -> ()  [unwired: 1 in, 1 out]
      n9 = shared-variable "RT CompactRIO Target\\RT_EPICS_Shared_Variables.lvlib\\2iddVELO:VP:Scanning"(w10) -> ()  [unwired: 1 in, 1 out]
    }
  }
  n10 = node-c288() -> (w9:T15)  [unwired: 4 in]
  n11 = while {
    i -> [w20]
    stop <- w21 stop-if-true
    # "Command  Loop"
    n12 = Wait Until Next ms Multiple(millisecond multiple=u32 50) -> ()  [unwired: 1 out]
    n13 = case shown="False" "Stop System (Careful!!)" {
      tunnel: [FALSE TRUE] -> w21
      frame False {
        n14 = shared-variable "RT CompactRIO Target\\RT_EPICS_Shared_Variables.lvlib\\2iddVELO:VP:Remote_Scan"() -> (w32:bool, error out=w30:errorcluster)  [unwired: 1 in]
        n15 = shared-variable "RT CompactRIO Target\\RT_EPICS_Shared_Variables.lvlib\\2iddVELO:VP:Local_Lock"("Local_Lock", error in=w30) -> (error out=w25:errorcluster)
        n16 = shared-variable ".\\Interloop communication.lvlib\\New Command"() -> (w35:bool)  [unwired: 1 in, 1 out]
        n17 = Not(x="Local_Lock") -> (.not. x?=w27:bool)
        n18 = And(x=w32, y=w27) -> (x .and. y?=w33:bool)
        "Remote Mode" <- w33
        n19 = Not(x=w35) -> (.not. x?=w34:bool)
        n20 = case shown="False" w33 {
          tunnel: w34 -> [w45 w57]
          tunnel: [Local_or_Remote."Local Control" ("Local or EPICS") Local_or_Remote."EPICS Control" ("Local or EPICS")] -> w24
          tunnel: w25 -> [w39 w52]
          tunnel: [w41 w55] -> w29
          tunnel: ["Base name" w54] -> w26
          frame False {
            # "Running  in local mode"
            n21 = And(x="Execute", y=w45) -> (x .and. y?=w43:bool)
            n22 = case shown="True" w43 {
              frame False {
              }
              frame True {
                n23 = shared-variable ".\\Interloop communication.lvlib\\New Command"(TRUE ("New Command")) -> ()  [unwired: 1 in, 1 out]
                n24 = shared-variable ".\\Interloop communication.lvlib\\System command"("System command") -> ()  [unwired: 1 in, 1 out]
                n25 = local write "Execute"(FALSE ("Execute")) -> ()
              }
            }
            n26 = Format Into String(error in=w39, "Scan type") -> (resulting string=w40:string, error out=w38:errorcluster)  [unwired: 2 in]
            n27 = shared-variable "RT CompactRIO Target\\RT_EPICS_Shared_Variables.lvlib\\2iddVELO:VP:Scan_Type"(w40, error in=w38) -> (error out=w41:errorcluster)
          }
          frame True {
            # "Running in remote mode via EPICS PVs"
            n28 = shared-variable "RT CompactRIO Target\\RT_EPICS_Shared_Variables.lvlib\\2iddVELO:VP:Execute_Command"(error in=w52) -> (w53:bool, error out=w51:errorcluster)
            "EPICS Execute Command" <- w53
            n29 = shared-variable "RT CompactRIO Target\\RT_EPICS_Shared_Variables.lvlib\\2iddVELO:VP:Base_Filename"() -> (w54:string)  [unwired: 1 in, 1 out]
            n30 = And(x=w57, y=w53) -> (x .and. y?=w56:bool)
            n31 = case shown="True" w56 {
              tunnel: [w58 w68] -> w55
              tunnel: w51 -> [w58 w65]
              frame False {
              }
              frame True {
                n32 = local read "EPICS cRIO Command"() -> (w66:T14)
                n33 = local read "EPICS Scan Type"() -> (w62:T2)
                n34 = shared-variable "RT CompactRIO Target\\RT_EPICS_Shared_Variables.lvlib\\2iddVELO:VP:Execute_Command"(FALSE ("2iddVELO:VP:Flyscan_Start"), error in=w65) -> (error out=w68:errorcluster)
                n35 = shared-variable ".\\Interloop communication.lvlib\\New Command"(TRUE ("New Command")) -> ()  [unwired: 1 in, 1 out]
                n36 = case shown="\"Fly\", Default" w62 {
                  tunnel: [T7."Custom Up Down Ramp" ("X Reference Wave Selection") T7."Constant" ("X Reference Wave Selection")] -> w61
                  tunnel: [T8."Custom Ramp Wave" ("Y Reference Wave Selection") T8."Constant" ("Y Reference Wave Selection")] -> w60
                  tunnel: [T6."Sine Wave" ("Z Reference Wave Selection") T6."Constant" ("Z Reference Wave Selection")] -> w59
                  frame "Fly", Default {
                  }
                  frame "Step" {
                  }
                }
                n37 = case shown="\"Reload Controller\"" w66 {
                  tunnel: [Command_Enum."Scan" ("System command") Command_Enum."Stop Scan" ("System command") Command_Enum."Re-Initialize " ("System command")] -> w63
                  frame "Start Scan", Default {
                  }
                  frame "Stop Scan" {
                  }
                  frame "Reload Controller" {
                  }
                }
                n38 = local write "Scan type"(w62) -> ()
                n39 = local write "X Reference Wave Selection"(w61) -> ()
                n40 = local write "Y Reference Wave Selection"(w60) -> ()
                n41 = local write "Z Reference Wave Selection"(w59) -> ()
                n42 = shared-variable ".\\Interloop communication.lvlib\\System command"(w63) -> ()  [unwired: 1 in, 1 out]
                n43 = local write "System Loop Type"(enum16{"Open Loop", "Closed Loop"}."Closed Loop" ("System Loop Type")) -> ()
              }
            }
            n44 = local write "Base name"(w54) -> ()
            n45 = local read "EPICS Controller Type"() -> (w50:T3)
            n46 = local write "Controller Type"(w50) -> ()
          }
        }
        "Local or EPICS" <- w24
        "Command Loop Error" <- w29
        n47 = shared-variable ".\\Interloop communication.lvlib\\Base Filename"(w26) -> ()  [unwired: 1 in, 1 out]
        n48 = shared-variable ".\\Interloop communication.lvlib\\Command Loop Error"(w29) -> ()  [unwired: 1 in, 1 out]
      }
      frame True {
        n49 = shared-variable ".\\Interloop communication.lvlib\\System command"(Command_Enum."Stop System" ("System command")) -> (error out=w79:errorcluster)  [unwired: 1 in]
        n50 = shared-variable ".\\Interloop communication.lvlib\\New Command"(TRUE ("New Command"), error in=w79) -> ()  [unwired: 1 out]
      }
    }
    "Command Loop Iterations" <- w20
  }
  n51 = while {
    shift-right: [w96] -> _
    shift-left: TRUE -> [w97]
    i -> [w85]
    stop <- w89 stop-if-true
    # "Heartbeat Loop"
    n52 = shared-variable ".\\Interloop communication.lvlib\\EPICS command error"() -> (w83:errorcluster)  [unwired: 1 in, 1 out]
    n53 = shared-variable ".\\Interloop communication.lvlib\\Command Loop Error"() -> (w91:errorcluster)  [unwired: 1 in, 1 out]
    n54 = shared-variable ".\\Interloop communication.lvlib\\FPGA startup error"() -> (w88:errorcluster)  [unwired: 1 in, 1 out]
    n55 = Not(x=w97) -> (.not. x?=w96:bool)
    "Heartbeat" <- w96
    n56 = shared-variable ".\\Interloop communication.lvlib\\Readback Loop Error"() -> (w90:errorcluster)  [unwired: 1 in, 1 out]
    n57 = shared-variable ".\\Interloop communication.lvlib\\Main Loop Error"() -> (w95:errorcluster)  [unwired: 1 in, 1 out]
    n58 = call <vilib>:"RT LEDs.vi"("State"=3, "LED Num"=0) -> ("error out"=w84:errorcluster)  [unwired: 4 in, 1 out]
    n59 = Merge Errors(w84, w83, w91, w88, w95, w90) -> (w92:errorcluster)
    n60 = case shown="No Error" w92 {
      selector: w92 -> [w98 w100]
      tunnel: [u32 500 ("millisecond multiple") u32 100 ("millisecond multiple")] -> w94
      tunnel: [w98 w100] -> w93
      frame No Error {
      }
      frame Error {
      }
    }
    "RT error" <- w93
    n61 = local read "Stop System (Careful!!)"() -> (w89:bool)
    n62 = Wait Until Next ms Multiple(millisecond multiple=w94) -> ()  [unwired: 1 out]
    "Heartbeat Loop Iterations" <- w85
  }
  n63 = timed-loop {
    timing: w9 -> [_]
    timing-out: [_] -> w8
    shift-right: [w109] -> _
    shift-left: w4 -> [w103]
    shift-right: [w116] -> _
    shift-left: w2 -> [w110]
    shift-right: [w107] -> _
    shift-left: w1 -> [w111]
    shift-right: [w113] -> _
    shift-left: w3 -> [w114]
    i -> [w115]
    stop <- w118 stop-if-true
    # "Main Loop"
    n64 = node-c288() -> ()  [unwired: 1 in, 1 out]
    n65 = Format Into String(format string="%s", w103) -> (resulting string=w104:string)  [unwired: 2 in, 1 out]
    n66 = local read "Local or EPICS"() -> (w108:T11)
    n67 = shared-variable "RT CompactRIO Target\\RT_EPICS_Shared_Variables.lvlib\\2iddVELO:VP:RT_State"(w104) -> ()  [unwired: 1 in, 1 out]
    n68 = local read "Scan type"() -> (w102:T2)
    n69 = case shown="\"Wait\"" w103 {
      tunnel: [w125 w145 w183 w241 w284 w398 w431 w444 w467 w503 w528 w567 w618 w646 w658] -> w117
      tunnel: [FALSE ("Stop") FALSE ("Stop") FALSE ("Stop") FALSE ("Stop") FALSE ("Stop") FALSE ("Stop") FALSE ("Stop") FALSE ("Stop") _ FALSE ("Stop") FALSE ("Stop") FALSE ("Stop") FALSE ("Stop") FALSE ("Stop") TRUE ("Stop")] -> w118
      tunnel: [w128 w150 w182 w243 w282 w397 w430 w446 w458 w495 w521 w588 w605 w641 w655] -> w116
      tunnel: [w120 w147 w181 w237 w281 w396 w429 w437 w457 w498 w520 w586 w617 w640 w660] -> w107
      tunnel: w111 -> [w126 w142 w185 w238 w290 w400 w432 w447 w465 w496 w522 w593 w610 w644 w664]
      tunnel: w110 -> [w127 w150 w184 w243 w291 w401 w433 w448 w466 w494 w523 w589 w612 w650 w665]
      tunnel: w114 -> [w125 w145 w183 _ w284 w398 w431 w444 w467 w503 w529 w568 w618 w646 _]
      tunnel: [i64 0 i64 0 i64 0 i64 50 i64 0 i64 0 i64 0 i64 0 i64 0 i64 250 i64 50 w553 i64 0 i64 0 i64 0] -> w112
      tunnel: w108 -> [_ _ _ _ w278 w393 _ _ _ _ w516 _ _ _ _]
      tunnel: w102 -> [_ _ _ w235 w277 _ _ _ _ w493 _ _ w607 _ _]
      frame "Initialization", Default {
        n70 = xnode "Invoke Method"("FPGA VI Reference In"=w127, "error in"=w126, "Requested Depth"="Requested Depth") -> ("FPGA VI Reference Out"=w130:refnum<k20>, "error out"=w129:errorcluster, "Actual Depth"=→"Actual Depth":u32)
        n71 = xnode "Read/Write Control"("FPGA VI Reference In"=w130, "error in"=w129, "Datalog Time Period (uSec)"="Datalog Time Period (uSec)", "Datalog Cases"="Datalog Cases") -> ("FPGA VI Reference Out"=w122:refnum<k20>, "error out"=w121:errorcluster)
        n72 = xnode "Read/Write Control"("FPGA VI Reference In"=w122, "error in"=w121) -> ("FPGA VI Reference Out"=w128:refnum<k20>, "error out"=w120:errorcluster, "Wait error"=w119:errorcluster)
        "FPGA wait error" <- w119
        n73 = shared-variable ".\\Interloop communication.lvlib\\FPGA startup error"(w119) -> ()  [unwired: 1 in, 1 out]
      }
      frame "Import Controller coeffs" {
        n74 = case shown="\"PID\"" "Controller Type" {
          tunnel: ["file path soscoeff_xx1 Hinf" "file path soscoeff_xx1 PID"] -> w141
          tunnel: ["file path sos gain SF Controller_xx1 Hinf" "file path sos gain SF Controller_xx1 PID"] -> w140
          tunnel: ["file path soscoeff_yy1 Hinf" "file path soscoeff_yy1 PID"] -> w139
          tunnel: ["file path sos gain SF Controller_yy1 Hinf" "file path sos gain SF Controller_yy1 PID"] -> w138
          tunnel: ["file path sos gain SF Controller_zz1 Hinf" "file path sos gain SF Controller_zz1 PID"] -> w137
          tunnel: ["file path soscoeff_zz1 Hinf" "file path soscoeff_zz1 PID"] -> w136
          frame "H-infinity", Default {
          }
          frame "PID" {
          }
        }
        n75 = call "Read_coeff.vi"("error in (no error)"=w142, "sos gain SF controller file path"=w137, "sos coeff file path"=w136) -> ("b02(2)"=→"b02(2) zz1c":fxp<+/-,64,9>[], "b01(2)"=→"b01(2) zz1c":fxp<+/-,64,9>[], "-a02(2)"=→"-a02(2) zz1c":fxp<+/-,64,9>[], "-a01(2)"=→"-a01(2) zz1c":fxp<+/-,64,9>[], "error out"=w146:errorcluster, "sos gain SF Controller"=→"sos gain SF Controller zz1c":fxp<+/-,42,9>)  [unwired: 3 in]
        n76 = call "Read_coeff.vi"("error in (no error)"=w142, "sos gain SF controller file path"=w138, "sos coeff file path"=w139) -> ("b02(2)"=→"b02(2) yy1c":fxp<+/-,64,9>[], "b01(2)"=→"b01(2) yy1c":fxp<+/-,64,9>[], "-a02(2)"=→"-a02(2) yy1c":fxp<+/-,64,9>[], "-a01(2)"=→"-a01(2) yy1c":fxp<+/-,64,9>[], "error out"=w144:errorcluster, "sos gain SF Controller"=→"sos gain SF Controller yy1c":fxp<+/-,42,9>)  [unwired: 3 in]
        n77 = call "Read_coeff.vi"("error in (no error)"=w142, "sos gain SF controller file path"=w140, "sos coeff file path"=w141) -> ("b02(2)"=→"b02(2) xx1c":fxp<+/-,64,9>[], "b01(2)"=→"b01(2) xx1c":fxp<+/-,64,9>[], "-a02(2)"=→"-a02(2) xx1c":fxp<+/-,64,9>[], "-a01(2)"=→"-a01(2) xx1c":fxp<+/-,64,9>[], "error out"=w143:errorcluster, "sos gain SF Controller"=→"sos gain SF Controller xx1c":fxp<+/-,42,9>)  [unwired: 3 in]
        n78 = Merge Errors(w143, w144, w146) -> (w147:errorcluster)
        "Coeff file import error" <- w147
      }
      frame "Update Controller Info" {
        n79 = local read "sos gain SF Controller yy1c"() -> (w214:fxp<+/-,42,9>)
        n80 = local read "sos gain SF Controller xx1c"() -> (w219:fxp<+/-,42,9>)
        n81 = local read "sos gain SF Controller zz1c"() -> (w212:fxp<+/-,42,9>)
        n82 = local read "-a01(2) yy1c"() -> (w218:fxp<+/-,64,9>[])
        n83 = local read "-a02(2) yy1c"() -> (w217:fxp<+/-,64,9>[])
        n84 = local read "-a01(2) xx1c"() -> (w223:fxp<+/-,64,9>[])
        n85 = local read "-a02(2) xx1c"() -> (w222:fxp<+/-,64,9>[])
        n86 = local read "-a01(2) zz1c"() -> (w213:fxp<+/-,64,9>[])
        n87 = local read "-a02(2) zz1c"() -> (w209:fxp<+/-,64,9>[])
        n88 = local read "b01(2) yy1c"() -> (w216:fxp<+/-,64,9>[])
        n89 = local read "b02(2) yy1c"() -> (w215:fxp<+/-,64,9>[])
        n90 = local read "b01(2) xx1c"() -> (w221:fxp<+/-,64,9>[])
        n91 = local read "b02(2) xx1c"() -> (w220:fxp<+/-,64,9>[])
        n92 = local read "b01(2) zz1c"() -> (w210:fxp<+/-,64,9>[])
        n93 = local read "b02(2) zz1c"() -> (w211:fxp<+/-,64,9>[])
        n94 = Or(x="Optics Z Reset", y="Reset All") -> (x .or. y?=w203:bool)
        n95 = Or(x="Sample Z Reset", y="Reset All") -> (x .or. y?=w200:bool)
        n96 = Or(x="Optics X Reset", y="Reset All") -> (x .or. y?=w207:bool)
        n97 = Or(x="Optics Y Reset", y="Reset All") -> (x .or. y?=w205:bool)
        n98 = Or(x="Sample X Reset", y="Reset All") -> (x .or. y?=w202:bool)
        n99 = Or(x="Sample Y Reset", y="Reset All") -> (x .or. y?=w201:bool)
        n100 = xnode "Read/Write Control"("FPGA VI Reference In"=w184, "error in"=w185, "Wait timer (ms)"="FPGA Wait Timer (ms)", "Controller Time Period (uSec)"="Controller Time Period (uSec)", "Controller Output Time Period (uSec)"="Controller Output Time Period (uSec)", "System Loop Type"="System Loop Type", "Controller Output Upper Limit"="Controller Output Upper Limit", "Controller Output Lower Limit"="Controller Output Lower Limit", "X-Stage nm to V Scaling"="X-Stage nm to V Scaling", "X-Stage Scaling Direction"="X-Stage Scaling Direction", "Y-Stage nm to V Scaling"="Y-Stage nm to V Scaling", "Z-Stage nm to V Scaling"="Z-Stage nm to V Scaling", "Plant Output Time Period (uSec)"="Plant Output Time Period (uSec)", "Reset Optics X"=w207, "Reset Optics Y"=w205, "Reset Optics Z"=w203, "Reset Sample X"=w202, "Reset Sample Y"=w201, "Reset Sample Z"=w200, "Optics X Stage Resolution (nm)"="Optics X Stage Resolution (nm)", "Optics Y Stage Resolution (nm)"="Optics Y Stage Resolution (nm)", "Optics Z Stage Resolution (nm)"="Optics Z Stage Resolution (nm)", "Sample X Stage Resolution (nm)"="Sample X Stage Resolution (nm)", "Sample Y Stage Resolution (nm)"="Sample Y Stage Resolution (nm)", "Sample Z Stage Resolution (nm)"="Sample Z Stage Resolution (nm)", "Scaling mV to V"="Scaling mV to V", "-a01(2) xx1"=w223, "-a02(2) xx1"=w222, "b01(2) xx1"=w221, "b02(2) xx1"=w220, "sos gain SF Controller xx1"=w219, "-a01(2) yy1"=w218, "-a02(2) yy1"=w217, "b01(2) yy1"=w216, "b02(2) yy1"=w215, "sos gain SF Controller yy1"=w214, "-a01(2) zz1"=w213, "-a02(2) zz1"=w209, "b01(2) zz1"=w210, "b02(2) zz1"=w211, "sos gain SF Controller zz1"=w212, "Analog Input Time Period (uSec)"="Analog Input Time Period (uSec)", "Optics and or Sample Stage"="Optics and or Sample Stage", "Y-Stage Scaling Direction"="Y-Stage Scaling Direction", "Z-Stage Scaling Direction"="Z-Stage Scaling Direction") -> ("FPGA VI Reference Out"=w182:refnum<k20>, "error out"=w181:errorcluster)
      }
      frame "Wait" {
        n101 = shared-variable ".\\Interloop communication.lvlib\\New Command"() -> (w242:bool, error out=w240:errorcluster)  [unwired: 1 in]
        n102 = case shown="True" w242 {
          tunnel: [w245 w247] -> w241
          tunnel: w240 -> [_ w251]
          tunnel: w238 -> [w244 w249]
          tunnel: [w244 w248] -> w237
          tunnel: w235 -> [_ w246]
          frame False {
            w245 = T13[] [enum."Wait"] items=["Initialization", "Import Controller coeffs", "Update Controller Info", "Wait", "Update Reference Info", "Update Detector Trigger Info", "Update Datalog Info", "Check FPGA Status", "Pre-Scan", "Start Scan", "Step Scanning", "Fly Scanning", "End Scan", "Restart FPGA", "Stop FPGA"]
          }
          frame True {
            n103 = shared-variable ".\\Interloop communication.lvlib\\System command"() -> (w250:T9)  [unwired: 1 in, 1 out]
            "Last Command Executed" <- w250
            n104 = case shown="\"Scan\"" w250 {
              tunnel: [w255 w258 w262 w267 w270 w274] -> w247
              tunnel: w249 -> [w254 w257 w261 w266 w269 w273]
              tunnel: [w253 w256 w260 w265 w268 w272] -> w248
              tunnel: w246 -> [_ _ w259 _ _ _]
              frame "Re-Initialize ", Default {
                w255 = T13[] [enum."Initialization", enum."Import Controller coeffs", enum."Update Controller Info", enum."Wait"] items=["Initialization", "Import Controller coeffs", "Update Controller Info", "Wait", "Update Reference Info", "Update Detector Trigger Info", "Update Datalog Info", "Check FPGA Status", "Pre-Scan", "Start Scan", "Step Scanning", "Fly Scanning", "End Scan", "Restart FPGA", "Stop FPGA"]
                n105 = call <vilib>:"Clear Errors.vi"("error in (no error)"=w254) -> ("error out"=w253:errorcluster)  [unwired: 5 in, 1 out]
              }
              frame "Update Scan Settings" {
                w258 = T13[] [enum."Update Reference Info", enum."Update Detector Trigger Info", enum."Update Datalog Info", enum."Wait"] items=["Initialization", "Import Controller coeffs", "Update Controller Info", "Wait", "Update Reference Info", "Update Detector Trigger Info", "Update Datalog Info", "Check FPGA Status", "Pre-Scan", "Start Scan", "Step Scanning", "Fly Scanning", "End Scan", "Restart FPGA", "Stop FPGA"]
                n106 = call <vilib>:"Clear Errors.vi"("error in (no error)"=w257) -> ("error out"=w256:errorcluster)  [unwired: 5 in, 1 out]
              }
              frame "Scan" {
                n107 = case shown="\"Fly\", Default" w259 {
                  tunnel: [w263 w264] -> w262
                  frame "Fly", Default {
                    w263 = T13[] [enum."Update Reference Info", enum."Update Detector Trigger Info", enum."Update Datalog Info", enum."Pre-Scan", enum."Start Scan", enum."Fly Scanning", enum."End Scan", enum."Wait"] items=["Initialization", "Import Controller coeffs", "Update Controller Info", "Wait", "Update Reference Info", "Update Detector Trigger Info", "Update Datalog Info", "Check FPGA Status", "Pre-Scan", "Start Scan", "Step Scanning", "Fly Scanning", "End Scan", "Restart FPGA", "Stop FPGA"]
                  }
                  frame "Step" {
                    w264 = T13[] [enum."Update Reference Info", enum."Update Detector Trigger Info", enum."Update Datalog Info", enum."Pre-Scan", enum."Start Scan", enum."Step Scanning", enum."End Scan", enum."Wait"] items=["Initialization", "Import Controller coeffs", "Update Controller Info", "Wait", "Update Reference Info", "Update Detector Trigger Info", "Update Datalog Info", "Check FPGA Status", "Pre-Scan", "Start Scan", "Step Scanning", "Fly Scanning", "End Scan", "Restart FPGA", "Stop FPGA"]
                  }
                }
                n108 = call <vilib>:"Clear Errors.vi"("error in (no error)"=w261) -> ("error out"=w260:errorcluster)  [unwired: 5 in, 1 out]
              }
              frame "Stop Scan" {
                w267 = T13[] [enum."End Scan", enum."Wait"] items=["Initialization", "Import Controller coeffs", "Update Controller Info", "Wait", "Update Reference Info", "Update Detector Trigger Info", "Update Datalog Info", "Check FPGA Status", "Pre-Scan", "Start Scan", "Step Scanning", "Fly Scanning", "End Scan", "Restart FPGA", "Stop FPGA"]
                n109 = call <vilib>:"Clear Errors.vi"("error in (no error)"=w266) -> ("error out"=w265:errorcluster)  [unwired: 5 in, 1 out]
              }
              frame "Restart FPGA" {
                w270 = T13[] [enum."Restart FPGA", enum."Initialization", enum."Import Controller coeffs", enum."Update Controller Info", enum."Wait"] items=["Initialization", "Import Controller coeffs", "Update Controller Info", "Wait", "Update Reference Info", "Update Detector Trigger Info", "Update Datalog Info", "Check FPGA Status", "Pre-Scan", "Start Scan", "Step Scanning", "Fly Scanning", "End Scan", "Restart FPGA", "Stop FPGA"]
                n110 = call <vilib>:"Clear Errors.vi"("error in (no error)"=w269) -> ("error out"=w268:errorcluster)  [unwired: 5 in, 1 out]
              }
              frame "Stop System" {
                w274 = T13[] [enum."Stop FPGA"] items=["Initialization", "Import Controller coeffs", "Update Controller Info", "Wait", "Update Reference Info", "Update Detector Trigger Info", "Update Datalog Info", "Check FPGA Status", "Pre-Scan", "Start Scan", "Step Scanning", "Fly Scanning", "End Scan", "Restart FPGA", "Stop FPGA"]
                n111 = call <vilib>:"Clear Errors.vi"("error in (no error)"=w273) -> ("error out"=w272:errorcluster)  [unwired: 5 in, 1 out]
                n112 = local write "Stop System (Careful!!)"(TRUE ("Stop")) -> ()
              }
            }
            n113 = shared-variable ".\\Interloop communication.lvlib\\New Command"(FALSE ("New Command"), error in=w251) -> ()  [unwired: 1 out]
          }
        }
      }
      frame "Update Reference Info" {
        w343 = errorcluster {"status"=FALSE, "code"=0, "source"=""}  # error in (no error)
        w346 = errorcluster {"status"=FALSE, "code"=0, "source"=""}  # error in (no error)
        w360 = errorcluster {"status"=FALSE, "code"=0, "source"=""}  # error in (no error)
        w339 = 40000000.0  # FPGA clock rate (Hz)
        n114 = local read "Measured Z Reference Time Period (Ticks)"() -> (w283:u32)
        n115 = case shown="\"EPICS Control\"" w278 {
          tunnel: ["X Ramp Start (nm)" w376] -> w298
          tunnel: ["X Ramp End (nm)" w375] -> w297
          tunnel: ["Y Ramp Start (nm)" w374] -> w296
          tunnel: ["Y Ramp End (nm)" w373] -> w295
          tunnel: ["Y Step Size (nm)" w377] -> w294
          tunnel: ["X Step Size (nm)" w380] -> w293
          tunnel: [w368 w378] -> w292
          tunnel: ["Y Step Size (nm)" w377] -> w289
          tunnel: ["X Ramp Start (nm)" w376] -> w288
          tunnel: ["X Ramp End (nm)" w375] -> w287
          tunnel: ["Y Ramp Start (nm)" w374] -> w286
          tunnel: ["Y Ramp End (nm)" w373] -> w285
          frame "Local Control", Default {
            n116 = local read "DT Frequency (Hz)"() -> (w368:dbl)
          }
          frame "EPICS Control" {
            w379 = fxp<+/-,16,16> 0.0 ("fixed-point type")
            n117 = shared-variable "RT CompactRIO Target\\RT_EPICS_Shared_Variables.lvlib\\2iddVELO:VP:Trigger_Freq_Hz"() -> (w378:dbl)  [unwired: 1 in, 1 out]
            "2iddVELO:VP:Trigger_Freq_Hz" <- w378
            n118 = shared-variable "RT CompactRIO Target\\RT_EPICS_Shared_Variables.lvlib\\2iddVELO:VP:Y_Step_Size_nm"() -> (w382:dbl)  [unwired: 1 in, 1 out]
            "2iddVELO:VP:Y_Step_Size_nm" <- w382
            n119 = shared-variable "RT CompactRIO Target\\RT_EPICS_Shared_Variables.lvlib\\2iddVELO:VP:X_Step_Size_nm"() -> (w381:dbl)  [unwired: 1 in, 1 out]
            "2iddVELO:VP:X_Step_Size_nm" <- w381
            n120 = shared-variable "RT CompactRIO Target\\RT_EPICS_Shared_Variables.lvlib\\2iddVELO:VP:Y_Start_nm"() -> (w383:dbl)  [unwired: 1 in, 1 out]
            n121 = shared-variable "RT CompactRIO Target\\RT_EPICS_Shared_Variables.lvlib\\2iddVELO:VP:Y_End_nm"() -> (w372:dbl)  [unwired: 1 in, 1 out]
            n122 = shared-variable "RT CompactRIO Target\\RT_EPICS_Shared_Variables.lvlib\\2iddVELO:VP:X_Start_nm"() -> (w385:dbl)  [unwired: 1 in, 1 out]
            "2iddVELO:VP:X_Start_nm" <- w385
            n123 = shared-variable "RT CompactRIO Target\\RT_EPICS_Shared_Variables.lvlib\\2iddVELO:VP:X_End_nm"() -> (w384:dbl)  [unwired: 1 in, 1 out]
            "2iddVELO:VP:X_End_nm" <- w384
            n124 = Negate(x=w372) -> (-x=w371:dbl)
            "2iddVELO:VP:Y_End_nm" <- w371
            n125 = Negate(x=w383) -> (-x=w370:dbl)
            "2iddVELO:VP:Y_Start_nm" <- w370
            n126 = To Fixed-Point(fixed-point type=w379, number=w385) -> (fixed-point=w376:fxp<+/-,16,16>)
            n127 = To Fixed-Point(fixed-point type=w379, number=w384) -> (fixed-point=w375:fxp<+/-,16,16>)
            n128 = To Fixed-Point(fixed-point type=w379, number=w370) -> (fixed-point=w374:fxp<+/-,16,16>)
            n129 = To Fixed-Point(fixed-point type=w379, number=w371) -> (fixed-point=w373:fxp<+/-,16,16>)
            n130 = To Fixed-Point(fixed-point type=w379, number=w382) -> (fixed-point=w377:fxp<+/-,16,16>)
            n131 = To Fixed-Point(fixed-point type=w379, number=w381) -> (fixed-point=w380:fxp<+/-,16,16>)
          }
        }
        n132 = Equal?(x=w277, y=Scan_type."Fly") -> (x = y?=w275:bool)
        n133 = local read "Y Ramp Period (usec)"() -> (w300:fxp<+,24,24>)
        n134 = case shown="\"Filtered White Noise\"" "Z Reference Wave Selection" {
          tunnel: "Z frequency (Hz)" -> [w386 w387 w389 w391 w392]
          tunnel: [w386 w387 w388 w391 w392] -> w321
          tunnel: w283 -> [_ _ w390 _ _]
          frame "Constant", Default {
          }
          frame "Sine Wave" {
          }
          frame "Sawtooth Wave" {
            n135 = Multiply(x=w390, y=w389) -> (x*y=w388:dbl)
          }
          frame "Square Wave" {
          }
          frame "Filtered White Noise" {
          }
        }
        n136 = call <vilib>:"Normalize Signal Generation Parameters.vi"("frequency (Hz)"="X frequency (Hz)", "FPGA clock rate (Hz)"=w339, "phase offset (deg)"="X phase offset (deg)", "error in (no error)"=w360) -> ("frequency (periods/tick)"=w359:fxp<+,32,0>, "phase offset (periods)"=w349:fxp<+,32,0>, "error out"=→"error out (Sig Gen)":errorcluster)  [unwired: 6 in, 3 out]
        "X frequency (periods/tick)" <- w359
        "X phase offset (periods)" <- w349
        n137 = call <vilib>:"Normalize Signal Generation Parameters.vi"("frequency (Hz)"="Y frequency (Hz)", "FPGA clock rate (Hz)"=w339, "phase offset (deg)"="Y phase offset (deg)", "error in (no error)"=w346) -> ("frequency (periods/tick)"=w342:fxp<+,32,0>, "phase offset (periods)"=w341:fxp<+,32,0>, "error out"=→"error out (Sig Gen) 2":errorcluster)  [unwired: 6 in, 3 out]
        "Y frequency (periods/tick)" <- w342
        "Y phase offset (periods)" <- w341
        n138 = call <vilib>:"Normalize Signal Generation Parameters.vi"("frequency (Hz)"=w321, "FPGA clock rate (Hz)"=w339, "phase offset (deg)"="Z phase offset (deg)", "error in (no error)"=w343) -> ("frequency (periods/tick)"=w340:fxp<+,32,0>, "phase offset (periods)"=w332:fxp<+,32,0>, "error out"=→"error out (Sig Gen) 3":errorcluster)  [unwired: 6 in, 3 out]
        "Z frequency (periods/tick)" <- w340
        "Z phase offset (periods)" <- w332
        n139 = local read "X Ramp Period (usec)"() -> (w299:fxp<+,24,24>)
        n140 = xnode "Read/Write Control"("FPGA VI Reference In"=w291, "error in"=w290, "X Reference Time Period (uSec)"="X Reference Time Period (uSec)", "Y Reference Time Period (uSec)"="Y Reference Time Period (uSec)", "Z Reference Time Period (uSec)"="Z Reference Time Period (uSec)", "X Reference Wave Selection"="X Reference Wave Selection", "Y Reference Wave Selection"="Y Reference Wave Selection", "Z Reference Wave Selection"="Z Reference Wave Selection", "X Reference Reset"="X Reference Reset", "Y Reference Reset"="Y Reference Reset", "Z Reference Reset"="Z Reference Reset", "X Reference Amplitude (nm)"="X Reference Amplitude (nm)", "Y Reference Amplitude (nm)"="Y Reference Amplitude (nm)", "Z Reference Amplitude (nm)"="Z Reference Amplitude (nm)", "X Frequency (periods/tick)"=w359, "X Phase Offset (periods)"=w349, "Y Frequency (periods/tick)"=w342, "Y Phase Offset (periods)"=w341, "Z Frequency (periods/tick)"=w340, "Z Phase Offset (periods)"=w332, "X Reference DC Offset (nm)"="X Reference DC Offset (nm)", "Y Reference DC Offset (nm)"="Y Reference DC Offset (nm)", "Z Reference DC Offset (nm)"="Z Reference DC Offset (nm)", "X White Noise Amplitude"="X White Noise Amplitude", "X White Noise Seed"="X White Noise Seed", "Y White Noise Amplitude"="Y White Noise Amplitude", "Y White Noise Seed"="Y White Noise Seed", "Z White Noise Amplitude"="Z White Noise Amplitude", "Z White Noise Seed"="Z White Noise Seed", "Mod 3 AI0 V to nm Scaling"="Mod 3 AI0 V to nm Scaling", "Mod 3 AI1 V to nm Scaling"="Mod 3 AI1 V to nm Scaling", "Mod 3 AI2 V to nm Scaling"="Mod 3 AI2 V to nm Scaling", "X Ramp Period (usec)"=w299, "X Ramp Start (nm)"=w298, "X Ramp End (nm)"=w297, "X Start Marker (nm)"="X Start Marker (nm)", "Fly Scan"=w275, "Y Ramp Period (usec)"=w300, "Y Ramp Start (nm)"=w296, "Y Ramp End (nm)"=w295, "Y Ramp Drop Size (nm)"=w294, "Y Start Marker (nm)"="Y Start Marker (nm)") -> ("FPGA VI Reference Out"=w282:refnum<k20>, "error out"=w281:errorcluster)
        n141 = Subtract(x=w286, y=w285) -> (x-y=w316:fxp<+/-,17,17>)
        n142 = Subtract(x=w288, y=w287) -> (x-y=w314:fxp<+/-,17,17>)
        n143 = Absolute Value(x=w316) -> (abs(x)=w307:fxp<+,16,16>)
        n144 = Absolute Value(x=w314) -> (abs(x)=w313:fxp<+,16,16>)
        n145 = Divide(x=w313, y=w293) -> (x/y=w311:fxp<+/-,33,17>)
        "# of Points per Line" <- w311
        n146 = Divide(x=w311, y=w292) -> (x/y=w303:dbl)
        "sec per line" <- w303
        n147 = Divide(x=w307, y=w289) -> (x/y=w308:fxp<+/-,33,17>)
        n148 = Add(x=w308, y=fxp<+,16,16> 1.0) -> (x+y=w302:fxp<+/-,34,18>)
        "# of Hor Lines" <- w302
        n149 = Multiply(x=w303, y=1000000.0) -> (x*y=w306:dbl)
        "X Ramp Period DBL (usec)" <- w306
        n150 = Reciprocal(x=w303) -> (1/x=→"line per sec (Hz)":dbl)
        n151 = To Fixed-Point(fixed-point type=fxp<+,24,24> 0.0, number=w306) -> (fixed-point=→"X Ramp Period (usec)" →"Y Ramp Period (usec)":fxp<+,24,24>)
        n152 = Multiply(x=w303, y=w302) -> (x*y=→"Total Scan Time (sec)":dbl)
        n153 = Multiply(x=w302, y=w311) -> (x*y=→"# Total Trigger Points":fxp<+/-,64,34>)
      }
      frame "Update Detector Trigger Info" {
        w407 = 40000000.0  # FPGA clock rate (Hz)
        w409 = errorcluster {"status"=FALSE, "code"=0, "source"=""}  # error in (no error)
        n154 = case shown="\"EPICS Control\"" w393 {
          tunnel: ["DT Frequency (Hz)" w426] -> w408
          tunnel: ["DT duty cycle (%)" w425] -> w402
          frame "Local Control", Default {
          }
          frame "EPICS Control" {
            n155 = shared-variable "RT CompactRIO Target\\RT_EPICS_Shared_Variables.lvlib\\2iddVELO:VP:Trig_DutyCycle_Per"() -> (w425:dbl)  [unwired: 1 in, 1 out]
            "2iddVELO:VP:Trig_DutyCycle_Per" <- w425
            n156 = shared-variable "RT CompactRIO Target\\RT_EPICS_Shared_Variables.lvlib\\2iddVELO:VP:Trigger_Freq_Hz"() -> (w426:dbl)  [unwired: 1 in, 1 out]
          }
        }
        "Trigger Frequency (Hz)" <- w408
        "Trigger Duty Cycle (%)" <- w402
        n157 = call <vilib>:"Normalize Signal Generation Parameters.vi"("frequency (Hz)"=w408, "FPGA clock rate (Hz)"=w407, "phase offset (deg)"="DT phase offset (deg)", "duty cycle (%)"=w402, "error in (no error)"=w409) -> ("frequency (periods/tick)"=w405:fxp<+,32,0>, "phase offset (periods)"=w404:fxp<+,32,0>, "duty cycle (periods)"=w403:fxp<+,32,0>, "error out"=→"error out (Sig Gen) 4":errorcluster)  [unwired: 5 in, 2 out]
        "DT Frequency (periods/tick)" <- w405
        "DT Phase Offset (periods)" <- w404
        "DT Duty Cycle (periods)" <- w403
        n158 = xnode "Read/Write Control"("FPGA VI Reference In"=w401, "error in"=w400, "Detector Trigger Time Period (uSec)"="Detector Trigger Time Period (uSec)", "Trigger Generation Time Period (uSec)"="Trigger Generation Time Period (uSec)", "Detector Trigger Lower Limit (V)"="Detector Trigger Lower Limit (V)", "Detector Trigger Upper Limit (V)"="Detector Trigger Upper Limit (V)", "Trigger High Period (usec)"="Trigger High Period (usec)", "Trigger Low Period (usec)"="Trigger Low Period (usec)", "Trigger High Level (V)"="Trigger High Level (V)", "Trigger Low Level (V)"="Trigger Low Level (V)", "Trigger Wave Generator"="Trigger Wave Generator", "DT Reference Amplitude (V)"="DT Reference Amplitude (V)", "DT Reference DC Offset (V)"="DT Reference DC Offset (V)", "DT Frequency (periods/tick)"=w405, "DT Phase Offset (periods)"=w404, "DT Reset"="DT Reset", "DT Duty Cycle (periods)"=w403, "Data Trigger Time Period (uSec)"="Data Trigger Time Period (uSec)") -> ("FPGA VI Reference Out"=w397:refnum<k20>, "error out"=w396:errorcluster)
      }
      frame "Update Datalog Info" {
        n159 = local read "Datalog Time Period (uSec)"() -> (w436:u32)
        n160 = local read "Datalog Cases"() -> (w435:T4)
        n161 = xnode "Read/Write Control"("FPGA VI Reference In"=w433, "error in"=w432, "Datalog Time Period (uSec)"=w436, "Datalog Cases"=w435, "Timeout FPGA FIFO1"="Timeout FPGA FIFO1") -> ("FPGA VI Reference Out"=w430:refnum<k20>, "error out"=w429:errorcluster)
      }
      frame "Check FPGA Status" {
        n162 = xnode "Read/Write Control"("FPGA VI Reference In"=w448, "error in"=w447) -> ("FPGA VI Reference Out"=w446:refnum<k20>, "error out"=w445:errorcluster, "FPGA error monitor"=w451:errorcluster, "End Run Error"=w450:errorcluster, "FIFO Timed Out?"=→"FIFO Timed Out?":bool, "stop case"=w440:bool, "FIFO Timed Out"=w441:bool)
        "FPGA error monitor" <- w451
        "FPGA end run error" <- w450
        "stop case" <- w440
        "FIFO Timed Out" <- w441
        n163 = case shown="True" w440 {
          tunnel: [errorcluster {"status"=FALSE, "code"=0, "source"=""} ("error constant") errorcluster {"status"=TRUE, "code"=7002, "source"="FPGA stop case encountered"} ("error constant")] -> w438
          frame False {
          }
          frame True {
          }
        }
        n164 = case shown="True" w441 {
          tunnel: [errorcluster {"status"=FALSE, "code"=0, "source"=""} ("error constant") errorcluster {"status"=TRUE, "code"=7001, "source"="FPGA FIFO timed out"} ("error constant")] -> w439
          frame False {
          }
          frame True {
          }
        }
        n165 = Merge Errors(w445, w451, w450, w438, w439) -> (w437:errorcluster)
      }
      frame "Pre-Scan" {
        n166 = flat-sequence {
          tunnel: w466 -> [w473]
          tunnel: w465 -> [w472]
          tunnel: [w469] -> w464
          tunnel: [w468] -> w462
          tunnel: w464 -> [w479]
          tunnel: [w479] -> w463
          tunnel: w462 -> [w478]
          tunnel: [w478] -> w461
          tunnel: w463 -> [w483]
          tunnel: w461 -> [w482]
          tunnel: [w481] -> w460
          tunnel: [w480] -> w459
          tunnel: w460 -> [w490]
          tunnel: w459 -> [w489]
          tunnel: [w486] -> w458
          tunnel: [w485] -> w457
          frame #0 {
            w470 = TRUE
            n167 = xnode "Read/Write Control"("FPGA VI Reference In"=w473, "error in"=w472, "Reset Optics X"=w470, "Reset Optics Y"=w470, "Reset Optics Z"=w470, "Reset Sample X"=w470, "Reset Sample Y"=w470, "Reset Sample Z"=w470, "System Loop Type"=enum16{"Open Loop", "Closed Loop"}."Open Loop", "New FPGA command"=TRUE, "FPGA command"=enum16{"Start Scan", "Shutdown"}."Start Scan", "Fly Scan"=FALSE) -> ("FPGA VI Reference Out"=w469:refnum<k20>, "error out"=w468:errorcluster)
          }
          frame #1 {
            n168 = Wait (ms)(milliseconds to wait="Pre-Scan pause (ms)") -> ()  [unwired: 1 out]
          }
          frame #2 {
            n169 = xnode "Read/Write Control"("FPGA VI Reference In"=w483, "error in"=w482, "stop case"=TRUE) -> ("FPGA VI Reference Out"=w481:refnum<k20>, "error out"=w480:errorcluster)
          }
          frame #3 {
            w487 = FALSE ("Reset Optics X")
            n170 = local read "System Loop Type"() -> (w488:enum16{"Open Loop", "Closed Loop"})
            n171 = xnode "Read/Write Control"("FPGA VI Reference In"=w490, "error in"=w489, "Reset Optics X"=w487, "Reset Optics Y"=w487, "Reset Optics Z"=w487, "Reset Sample X"=w487, "Reset Sample Y"=w487, "Reset Sample Z"=w487, "System Loop Type"=w488) -> ("FPGA VI Reference Out"=w486:refnum<k20>, "error out"=w485:errorcluster)
          }
        }
      }
      frame "Start Scan" {
        n172 = case shown="\"Fly\", Default" w493 {
          tunnel: [w506 w515] -> w497
          tunnel: w496 -> [w505 w515]
          tunnel: [TRUE ("2iddVELO:VP:Scanning") FALSE ("2iddVELO:VP:Scanning")] -> w491
          frame "Fly", Default {
            n173 = shared-variable ".\\Interloop communication.lvlib\\Base Filename"() -> (w507:string)  [unwired: 1 in, 1 out]
            n174 = String To Path(string="cRIO data dir") -> (path=w508:path)
            "cRIO path" <- w508
            n175 = call "Data_Write.vi"("Destination dir"=w508, "error initialize"=w505, "Base name"=w507, "Command List"=Data_Write_Control."Initialize") -> ("error out"=w506:errorcluster, "Path"=w512:path)  [unwired: 4 in]
            n176 = Strip Path(path=w512) -> (stripped path=→"Output path":path, name=→"Output filename":string)
          }
          frame "Step" {
          }
        }
        n177 = xnode "Read/Write Control"("FPGA VI Reference In"=w494, "error in"=w497, "New FPGA command"=TRUE, "FPGA command"=enum16{"Start Scan", "Shutdown"}."Start Scan", "Fly Scan"=w491) -> ("FPGA VI Reference Out"=w495:refnum<k20>, "error out"=w498:errorcluster)
        n178 = shared-variable "RT CompactRIO Target\\RT_EPICS_Shared_Variables.lvlib\\2iddVELO:VP:Scanning"(TRUE ("2iddVELO:VP:Scanning")) -> ()  [unwired: 1 in, 1 out]
      }
      frame "Step Scanning" {
        n179 = case shown="\"EPICS Control\"" w516 {
          tunnel: [w531 w533] -> w518
          tunnel: [w532 w536] -> w519
          tunnel: [w530 w534] -> w517
          frame "Local Control", Default {
            n180 = local read "X Reference Amplitude (nm)"() -> (w530:fxp<+/-,40,17>)
            n181 = local read "Y Reference Amplitude (nm)"() -> (w531:fxp<+/-,40,17>)
            n182 = local read "Z Reference Amplitude (nm)"() -> (w532:fxp<+/-,40,17>)
          }
          frame "EPICS Control" {
            w535 = fxp<+/-,40,17> 0.0 ("Z Reference Amplitude (nm)")
            n183 = shared-variable "RT CompactRIO Target\\RT_EPICS_Shared_Variables.lvlib\\2iddVELO:LabView:ZPZ_Command"() -> (w537:dbl)  [unwired: 1 in, 1 out]
            n184 = shared-variable "RT CompactRIO Target\\RT_EPICS_Shared_Variables.lvlib\\2iddVELO:LabView:ZPY_Command"() -> (w538:dbl)  [unwired: 1 in, 1 out]
            n185 = shared-variable "RT CompactRIO Target\\RT_EPICS_Shared_Variables.lvlib\\2iddVELO:LabView:ZPX_Command"() -> (w539:dbl)  [unwired: 1 in, 1 out]
            n186 = To Fixed-Point(fixed-point type=w535, number=w539) -> (fixed-point=w534:fxp<+/-,40,17>)
            n187 = To Fixed-Point(fixed-point type=w535, number=w538) -> (fixed-point=w533:fxp<+/-,40,17>)
            n188 = To Fixed-Point(fixed-point type=w535, number=w537) -> (fixed-point=w536:fxp<+/-,40,17>)
            n189 = local write "X Reference Amplitude (nm)"(w534) -> ()
            n190 = local write "Y Reference Amplitude (nm)"(w533) -> ()
            n191 = local write "Z Reference Amplitude (nm)"(w536) -> ()
          }
        }
        n192 = xnode "Read/Write Control"("FPGA VI Reference In"=w523, "error in"=w522, "X Reference Amplitude (nm)"=w517, "Y Reference Amplitude (nm)"=w518, "Z Reference Amplitude (nm)"=w519) -> ("FPGA VI Reference Out"=w521:refnum<k20>, "error out"=w520:errorcluster)
        n193 = Insert Into Array(array=w529, index=0, new element=State_Enum."Step Scanning" ("new element/subarray")) -> (w528:T13[])
      }
      frame "Fly Scanning" {
        w584 = "%8f"  # format string
        w583 = ","  # delimiter (Tab)
        w598 = 0.0  # t0
        # "This creates time gap between subsequent\n reads in order to fill FIFO to Number of Elements"
        n194 = xnode "Read/Write Control"("FPGA VI Reference In"=w589, "error in"=w593) -> ("FPGA VI Reference Out"=w578:refnum<k20>, "error out"=w577:errorcluster, "Number of Data Strings"=→"Number of Data Strings":i32, "FPGA state"=w573:T12)
        n195 = local read "Trigger Frequency (Hz)"() -> (w546:dbl)
        "Data Read Rate (Hz)" <- w546
        n196 = Not Equal?(x=T12."Run", y=w573) -> (x != y?=w570:bool)
        n197 = xnode "Invoke Method"("FPGA VI Reference In"=w578, "error in"=w577, "Number of Elements"=u32 0, "Timeout (ms)"=0) -> ("FPGA VI Reference Out"=w575:refnum<k20>, "error out"=w576:errorcluster, "Elements Remaining"=w552:u32)  [unwired: 1 out]
        "Elements Available in FIFO" <- w552
        n198 = Divide(x="FIFO Timeout (ms)", y=1000.0) -> (x/y=w542:dbl)
        n199 = Multiply(x=w542, y="FIFO Timeout ratio") -> (x*y=w544:dbl)
        n200 = Multiply(x=w544, y=w546) -> (x*y=w550:dbl)
        n201 = Multiply(x=w550, y=5.0) -> (x*y=w548:dbl)
        n202 = Multiply(x=i16 1000, y=w544) -> (x*y=w551:dbl)
        n203 = To Unsigned Long Integer(number=w548) -> (unsigned 32bit integer=w547:u32)
        "Number of Elements" <- w547
        n204 = Max & Min(x=w552, y=w547) -> (min(x,y)=w557:u32)  [unwired: 1 out]
        n205 = Equal?(x=u32 0, y=w552) -> (x = y?=w571:bool)
        n206 = And(x=w570, y=w571) -> (x .and. y?=w569:bool)
        n207 = xnode "Invoke Method"("FPGA VI Reference In"=w575, "error in"=w576, "Number of Elements"=w557, "Timeout (ms)"="FIFO Timeout (ms)") -> ("FPGA VI Reference Out"=w588:refnum<k20>, "error out"=w587:errorcluster, "Data"=w595:fxp<+/-,58,25>[], "Elements Remaining"=→"Elements Remaining" →"Elements Remaining in FIFO":u32)
        "Data" <- w595
        n208 = Reciprocal(x=w546) -> (1/x=w545:dbl)
        "Data Read Period (sec)" <- w545
        n209 = To Quad Integer(1:w551) -> (0:w553:i64)
        "Scan loop dt" <- w553
        n210 = Decimate 1D Array(w595) -> (w565:fxp<+/-,58,25>[], w564:fxp<+/-,58,25>[], w563:fxp<+/-,58,25>[], w562:fxp<+/-,58,25>[], w590:fxp<+/-,58,25>[])
        n211 = Build Array(w565, w564, w563, w562, w590) -> (w599:fxp<+/-,58,25>[][])
        n212 = To Double Precision Float(number=w599) -> (double precision float=w596:dbl[][])
        n213 = Transpose 2D Array(2D array=w596) -> (transposed array=w592:dbl[][])
        n214 = case shown="False" w569 {
          tunnel: w568 -> [w603 w604]
          tunnel: [w601 w604] -> w567
          frame False {
            # "Either FIFO not empty or FPGA not \ndone running -- repeat scanning state"
            n215 = Insert Into Array(array=w603, index=0, new element=State_Enum."Fly Scanning" ("new element/subarray")) -> (w601:T13[])
          }
          frame True {
            # "FIFO empty, FPGA done running \n-- moving onto next state"
          }
        }
        n216 = To Double Precision Float(number=w565) -> (double precision float=w561:dbl[])
        n217 = To Double Precision Float(number=w564) -> (double precision float=w560:dbl[])
        n218 = To Double Precision Float(number=w563) -> (double precision float=w559:dbl[])
        n219 = To Double Precision Float(number=w562) -> (double precision float=w558:dbl[])
        n220 = Bundle("t0"=w598, w545, w596) -> (→"Reference and Actual positions":cluster{"t0":dbl, dbl, dbl[][]})  [unwired: 1 in]
        n221 = Bundle(w559, w558) -> (→"XY actual":cluster{dbl[], dbl[]})  [unwired: 1 in]
        n222 = Bundle(w561, w560) -> (→"XY Ref":cluster{dbl[], dbl[]})  [unwired: 1 in]
        n223 = Array To Spreadsheet String(delimiter (Tab)=w583, array=w592, 3:w584) -> (spreadsheet string=w582:string)
        n224 = call "Data_Write.vi"("error initialize"=w593, "Data"=w582, "Command List"=Data_Write_Control."Write") -> ("error out"=w581:errorcluster)  [unwired: 5 in, 1 out]
        n225 = Merge Errors(w587, w581) -> (w586:errorcluster)
      }
      frame "End Scan" {
        n226 = case shown="\"Step\"" w607 {
          tunnel: w612 -> [w636 w637]
          tunnel: [w635 w637] -> w611
          tunnel: w610 -> [w634 w638]
          tunnel: [w633 w638] -> w609
          frame "Fly", Default {
            n227 = xnode "Invoke Method"("FPGA VI Reference In"=w636, "error in"=w634) -> ("FPGA VI Reference Out"=w635:refnum<k20>, "error out"=w633:errorcluster)
          }
          frame "Step" {
          }
        }
        n228 = xnode "Read/Write Control"("FPGA VI Reference In"=w611, "error in"=w609, "stop case"=TRUE ("New FPGA command")) -> ("FPGA VI Reference Out"=w606:refnum<k20>, "error out"=w614:errorcluster)
        n229 = shared-variable "RT CompactRIO Target\\RT_EPICS_Shared_Variables.lvlib\\2iddVELO:VP:Scanning"(FALSE ("2iddVELO:VP:Fly_Scanning")) -> ()  [unwired: 1 in, 1 out]
        n230 = case shown="\"Fly\", Default" w607 {
          tunnel: [w622 w631] -> w617
          tunnel: w614 -> [w621 w631]
          tunnel: w606 -> [w619 w632]
          tunnel: [w619 w632] -> w605
          frame "Fly", Default {
            n231 = call "Data_Write.vi"("error initialize"=w621, "Command List"=Data_Write_Control."Close") -> ("error out"=w620:errorcluster)  [unwired: 6 in, 1 out]
            n232 = case shown="No Error" w620 {
              tunnel: w620 -> [w629 w630]
              tunnel: [w628 w630] -> w622
              frame No Error {
                n233 = local read "Output filename"() -> (w624:string)
                n234 = local read "Output path"() -> (w625:path)
                n235 = Path To String(path=w625) -> (string=w627:string)
                n236 = shared-variable "RT CompactRIO Target\\RT_EPICS_Shared_Variables.lvlib\\2iddVELO:VP:Last_Filename"(w624, error in=w629) -> (error out=w626:errorcluster)
                n237 = shared-variable "RT CompactRIO Target\\RT_EPICS_Shared_Variables.lvlib\\2iddVELO:VP:cRIO_Dir"(w627, error in=w626) -> (error out=w628:errorcluster)
              }
              frame Error {
              }
            }
          }
          frame "Step" {
          }
        }
      }
      frame "Restart FPGA" {
        n238 = call <vilib>:"Clear Errors.vi"("error in (no error)"=w644) -> ("error out"=w645:errorcluster)  [unwired: 5 in, 1 out]
        n239 = xnode "Invoke Method"("FPGA VI Reference In"=w650, "error in"=w645) -> ("FPGA VI Reference Out"=w649:refnum<k20>, "error out"=w648:errorcluster)
        n240 = xnode "Read/Write Control"("FPGA VI Reference In"=w649, "error in"=w648, "stop case"=TRUE) -> ("FPGA VI Reference Out"=w643:refnum<k20>, "error out"=w642:errorcluster)
        n241 = xnode "Invoke Method"("FPGA VI Reference In"=w643, "error in"=w642) -> ("FPGA VI Reference Out"=w641:refnum<k20>, "error out"=w640:errorcluster)
      }
      frame "Stop FPGA" {
        w658 = T13[] [enum."Stop FPGA"] items=["Initialization", "Import Controller coeffs", "Update Controller Info", "Wait", "Update Reference Info", "Update Detector Trigger Info", "Update Datalog Info", "Check FPGA Status", "Pre-Scan", "Start Scan", "Step Scanning", "Fly Scanning", "End Scan", "Restart FPGA", "Stop FPGA"] ("Reduced Array of States")
        w657 = TRUE ("stop case")
        n242 = xnode "Invoke Method"("FPGA VI Reference In"=w665, "error in"=w664) -> ("FPGA VI Reference Out"=w663:refnum<k20>, "error out"=w662:errorcluster)
        n243 = xnode "Read/Write Control"("FPGA VI Reference In"=w663, "error in"=w662, "stop case"=w657, "New FPGA command"=w657, "FPGA command"=enum16{"Start Scan", "Shutdown"}."Shutdown") -> ("FPGA VI Reference Out"=w661:refnum<k20>, "error out"=w654:errorcluster)
        n244 = xnode "Invoke Method"("FPGA VI Reference In"=w661, "error in"=w654) -> ("FPGA VI Reference Out"=w655:refnum<k20>, "error out"=w653:errorcluster)
        n245 = xnode "Close FPGA VI Reference"("FPGA VI Reference In"=w655, "error in"=w653) -> ("error out"=w660:errorcluster)
      }
    }
    "Main Loop error" <- w107
    n246 = shared-variable ".\\Interloop communication.lvlib\\Main Loop Error"(w107) -> ()  [unwired: 1 in, 1 out]
    n247 = node-c288(w112) -> ()  [unwired: 1 out]
    n248 = call "State Control.vi"("Stop"=FALSE, "Array of States"=w117, "Error Input"=w107) -> ("Next State"=w109:T13, "Reduced Array of States"=w113:T13[])  [unwired: 5 in]
    "RT Main Loop State" <- w103
    "Main Loop Iterations" <- w115
    "Reduced Array of States" <- w114
  }
  n249 = while {
    tunnel: w2 -> [w674]
    tunnel: w1 -> [w673]
    i -> [w671]
    stop <- w672 stop-if-true
    # "Readback loop"
    n250 = local read "RT Main Loop State"() -> (w677:T13)
    n251 = Not Equal?(x=w677, y=State_Enum."Initialization") -> (x != y?=w675:bool)
    n252 = case shown="True" w675 {
      tunnel: w674 -> [_ w691]
      tunnel: w673 -> [_ w689]
      tunnel: [u32 100 ("milliseconds to wait") "Readback Loop time between iterations (ms)"] -> w670
      frame False {
      }
      frame True {
        w727 = 40000000.0  # FPGA Clock Rate (Hz)
        w746 = 40000000.0  # FPGA Clock Rate (Hz)
        w763 = 40000000.0  # FPGA Clock Rate (Hz)
        n253 = xnode "Read/Write Control"("FPGA VI Reference In"=w691, "error in"=w689) -> ("FPGA VI Reference Out"=w690:refnum<k20>, "error out"=w688:errorcluster, "FPGA state"=w685:T12, "Fly scan completed"=→"Fly Scan Complete":bool)
        "FPGA state" <- w685
        n254 = Format Into String(format string="%s", w685) -> (resulting string=w687:string)  [unwired: 2 in, 1 out]
        n255 = xnode "Read/Write Control"("FPGA VI Reference In"=w690, "error in"=w688) -> ("error out"=w697:errorcluster, "Measured Datalog Time Period (Ticks)"=w721:u32, "Measured Counter Time Period (Ticks)"=w726:u32, "Mod4/DIO0"=→"Mod4/DIO0":bool, "Mod4/DIO1"=→"Mod4/DIO1":bool, "Mod4/DIO2"=→"Mod4/DIO2":bool, "Mod4/DIO3"=→"Mod4/DIO3":bool, "Mod5/DIO0"=→"Mod5/DIO0":bool, "Mod5/DIO1"=→"Mod5/DIO1":bool, "Mod5/DIO2"=→"Mod5/DIO2":bool, "Mod5/DIO3"=→"Mod5/DIO3":bool, "Mod6/DIO0"=→"Mod6/DIO0":bool, "Mod6/DIO1"=→"Mod6/DIO1":bool, "Mod6/DIO2"=→"Mod6/DIO2":bool, "Mod6/DIO3"=→"Mod6/DIO3":bool, "32 bit Count Optics X"=→"32 bit Count Optics X":i32, "32 bit Count Optics  Y"=→"32 bit Count Optics  Y":i32, "32 bit Count Optics  Z"=→"32 bit Count Optics  Z":i32, "32 bit Count Sample X"=→"32 bit Count Sample X":i32, "32 bit Count Sample  Y"=→"32 bit Count Sample  Y":i32, "32 bit Count Sample  Z"=→"32 bit Count Sample  Z":i32, "Optics X Stage Displacement (nm)"=w684:fxp<+/-,58,25>, "Optics Y Stage Displacement (nm)"=w683:fxp<+/-,58,25>, "Optics Z Stage Displacement (nm)"=w682:fxp<+/-,58,25>, "Sample X Stage Displacement (nm)"=→"Sample X Stage Displacement (nm)":fxp<+/-,58,25>, "Sample Y Stage Displacement (nm)"=→"Sample Y Stage Displacement (nm)":fxp<+/-,58,25>, "Sample Z Stage Displacement (nm)"=→"Sample Z Stage Displacement (nm)":fxp<+/-,58,25>)  [unwired: 1 out]
        "Measured Datalog Time Period (Ticks)" <- w721
        "Measured Counter Time Period (Ticks)" <- w726
        "Optics X Stage Displacement (nm)" <- w684
        "Optics Y Stage Displacement (nm)" <- w683
        "Optics Z Stage Displacement (nm)" <- w682
        n256 = xnode "Read/Write Control"("FPGA VI Reference In"=w690, "error in"=w688) -> ("error out"=w696:errorcluster, "Measured Detector Trigger Time Period (Ticks)"=→"Measured Detector Trigger Time Period (Ticks)":u32, "Measured Trigger Gen Time Period (Ticks)"=→"Measured Trigger Gen Time Period (Ticks)":u32, "Detector Trigger (V)"=→"Detector Trigger (V)":fxp<+/-,20,5>, "Detector Trigger In Range?"=→"Detector Trigger In Range?":bool, "Measured Data Trigger Time Period (Ticks)"=→"Measured Data Trigger Time Period (Ticks)":u32, "Trigger for Data"=→"Trigger for Data":fxp<+/-,58,25>)  [unwired: 1 out]
        n257 = xnode "Read/Write Control"("FPGA VI Reference In"=w690, "error in"=w688) -> ("error out"=w694:errorcluster, "PI X-Stage Input (V)"=→"PI X-Stage Input (V)":fxp<+/-,20,5>, "PI Y-Stage Input (V)"=→"PI Y-Stage Input (V)":fxp<+/-,20,5>, "PI Z-Stage Input (V)"=→"PI Z-Stage Input (V)":fxp<+/-,20,5>, "X-Stage Input In Range?"=→"X-Stage Input In Range?":bool, "Y-Stage Input In Range?"=→"Y-Stage Input In Range?":bool, "Z-Stage Input In Range?"=→"Z-Stage Input In Range?":bool, "Measured Controller Time Period (Ticks)"=w767:u32, "Measured Controller Output Time Period (Ticks)"=w766:u32, "Measured Plant Output Time Period (Ticks)"=w765:u32, "Measured Analog Input Time Period (Ticks)"=w764:u32)  [unwired: 1 out]
        "Measured Controller Time Period (Ticks)" <- w767
        "Measured Controller Output Time Period (Ticks)" <- w766
        "Measured Plant Output Time Period (Ticks)" <- w765
        "Measured Analog Input Time Period (Ticks)" <- w764
        n258 = xnode "Read/Write Control"("FPGA VI Reference In"=w690, "error in"=w688) -> ("error out"=w695:errorcluster, "X Stage Reference (nm)"=→"X Stage Reference (nm)":fxp<+/-,58,25>, "Y Stage Reference (nm)"=→"Y Stage Reference (nm)":fxp<+/-,58,25>, "Z Stage Reference (nm)"=→"Z Stage Reference (nm)":fxp<+/-,58,25>, "Measured X Reference Time Period (Ticks)"=w748:u32, "Measured Y Reference Time Period (Ticks)"=w747:u32, "Measured Z Reference Time Period (Ticks)"=w739:u32, "Fly Scan Running"=→"Fly Scan Running":bool, "Continue Run"=→"Continue Run":bool)  [unwired: 1 out]
        "Measured X Reference Time Period (Ticks)" <- w748
        "Measured Y Reference Time Period (Ticks)" <- w747
        "Measured Z Reference Time Period (Ticks)" <- w739
        n259 = shared-variable "RT CompactRIO Target\\RT_EPICS_Shared_Variables.lvlib\\2iddVELO:VP:FPGA_State"(w687) -> ()  [unwired: 1 in, 1 out]
        n260 = call "Convert Measured Rate.vi"("FPGA Clock Rate (Hz)"=w746, "Measured Reference Time Period (Ticks)"=w739) -> ("Measured Reference Loop Rate (kHz)"=→"Measured Z Reference Loop Rate (kHz)":dbl, "Measured Reference Loop Period (s)"=→"Measured Z Reference Loop Rate (secs)":dbl)
        n261 = call "Convert Measured Rate.vi"("FPGA Clock Rate (Hz)"=w746, "Measured Reference Time Period (Ticks)"=w747) -> ("Measured Reference Loop Rate (kHz)"=→"Measured Y Reference Loop Rate (kHz)":dbl, "Measured Reference Loop Period (s)"=→"Measured Y Reference Loop Rate (secs)":dbl)
        n262 = call "Convert Measured Rate.vi"("FPGA Clock Rate (Hz)"=w727, "Measured Reference Time Period (Ticks)"=w726) -> ("Measured Reference Loop Rate (kHz)"=w724:dbl, "Measured Reference Loop Period (s)"=→"Measured Counter Loop Rate (secs)":dbl)
        n263 = call "Convert Measured Rate.vi"("FPGA Clock Rate (Hz)"=w746, "Measured Reference Time Period (Ticks)"=w748) -> ("Measured Reference Loop Rate (kHz)"=→"Measured X Reference Loop Rate (kHz)":dbl, "Measured Reference Loop Period (s)"=→"Measured X Reference Loop Rate (secs)":dbl)
        n264 = call "Convert Measured Rate.vi"("FPGA Clock Rate (Hz)"=w727, "Measured Reference Time Period (Ticks)"=w721) -> ("Measured Reference Loop Rate (kHz)"=→"Measured Datalog Loop Rate (kHz)":dbl, "Measured Reference Loop Period (s)"=→"Measured Datalog Loop Rate (secs)":dbl)
        n265 = call "Convert Measured Rate.vi"("FPGA Clock Rate (Hz)"=w763, "Measured Reference Time Period (Ticks)"=w767) -> ("Measured Reference Loop Rate (kHz)"=→"Measured Controller Loop Rate (kHz)":dbl, "Measured Reference Loop Period (s)"=→"Measured Controller Loop Rate (secs)":dbl)
        n266 = call "Convert Measured Rate.vi"("FPGA Clock Rate (Hz)"=w763, "Measured Reference Time Period (Ticks)"=w766) -> ("Measured Reference Loop Rate (kHz)"=→"Measured Controller Output Loop Rate (kHz)":dbl, "Measured Reference Loop Period (s)"=→"Measured Controller Output Loop Rate (secs)":dbl)
        n267 = call "Convert Measured Rate.vi"("FPGA Clock Rate (Hz)"=w763, "Measured Reference Time Period (Ticks)"=w765) -> ("Measured Reference Loop Rate (kHz)"=→"Measured Plant Output Loop Rate (kHz)":dbl, "Measured Reference Loop Period (s)"=→"Measured Plant Output Loop Rate (secs)":dbl)
        n268 = call "Convert Measured Rate.vi"("FPGA Clock Rate (Hz)"=w763, "Measured Reference Time Period (Ticks)"=w764) -> ("Measured Reference Loop Rate (kHz)"=→"Measured Analog Input Loop Rate (kHz)":dbl, "Measured Reference Loop Period (s)"=→"Measured Analog Input Loop Rate (secs)":dbl)
        n269 = Divide(x=w724, y=1000.0) -> (x/y=→"Measured Counter Loop Rate (MHz)":dbl)
        n270 = To Double Precision Float(number=w682) -> (double precision float=w679:dbl)
        n271 = To Double Precision Float(number=w684) -> (double precision float=w681:dbl)
        n272 = To Double Precision Float(number=w683) -> (double precision float=w680:dbl)
        n273 = shared-variable "RT CompactRIO Target\\RT_EPICS_Shared_Variables.lvlib\\2iddVELO:LabView:ZPY_Readback"(w680) -> ()  [unwired: 1 in, 1 out]
        n274 = shared-variable "RT CompactRIO Target\\RT_EPICS_Shared_Variables.lvlib\\2iddVELO:LabView:ZPX_Readback"(w681) -> ()  [unwired: 1 in, 1 out]
        n275 = shared-variable "RT CompactRIO Target\\RT_EPICS_Shared_Variables.lvlib\\2iddVELO:LabView:ZPZ_Readback"(w679) -> ()  [unwired: 1 in, 1 out]
        n276 = Merge Errors(w694, w695, w696, w697) -> (w693:errorcluster)
        "Readback error" <- w693
        n277 = shared-variable ".\\Interloop communication.lvlib\\Readback Loop Error"(w693) -> ()  [unwired: 1 in, 1 out]
      }
    }
    n278 = local read "Stop System (Careful!!)"() -> (w672:bool)
    n279 = Wait (ms)(milliseconds to wait=w670) -> ()  [unwired: 1 out]
    "Readback loop Iterations" <- w671
  }
  n280 = while {
    stop <- w785 stop-if-true
    n281 = shared-variable "RT CompactRIO Target\\RT_EPICS_Shared_Variables.lvlib\\2iddVELO:VP:Controller_Type"() -> (w783:string, error out=w774:errorcluster)  [unwired: 1 in]
    "2iddVELO:VP:Controller_Type" <- w783
    n282 = shared-variable "RT CompactRIO Target\\RT_EPICS_Shared_Variables.lvlib\\2iddVELO:VP:cRIO_Command"() -> (w782:string, error out=w776:errorcluster)  [unwired: 1 in]
    "2iddVELO:VP:cRIO_Command" <- w782
    n283 = shared-variable "RT CompactRIO Target\\RT_EPICS_Shared_Variables.lvlib\\2iddVELO:VP:Scan_Type"() -> (w780:string, error out=w772:errorcluster)  [unwired: 1 in]
    "2iddVELO:VP:Scan_Type" <- w780
    n284 = Scan From String(input string=w782, error in=w776, default 1=EPICS_Command_Control."Start Scan" ("default value 1")) -> (error out=w775:errorcluster, output 1=→"EPICS cRIO Command":T14)  [unwired: 2 in, 2 out]
    n285 = Scan From String(input string=w783, error in=w774, default 1=Controller_Type."H-infinity" ("Controller Type")) -> (error out=w773:errorcluster, output 1=→"EPICS Controller Type":T3)  [unwired: 2 in, 2 out]
    n286 = Scan From String(input string=w780, error in=w772, default 1=Scan_type."Fly" ("Scan type")) -> (error out=w771:errorcluster, output 1=→"EPICS Scan Type":T2)  [unwired: 2 in, 2 out]
    n287 = local read "Stop System (Careful!!)"() -> (w785:bool)
    n288 = Merge Errors(w775, w773, w771) -> (w770:errorcluster)
    "EPICS command error" <- w770
    n289 = shared-variable ".\\Interloop communication.lvlib\\EPICS command error"(w770) -> ()  [unwired: 1 in, 1 out]
    n290 = Wait Until Next ms Multiple(millisecond multiple=u32 100) -> ()  [unwired: 1 out]
  }
  n291 = node-c288(w8) -> (→"Timed Loop (end error)":errorcluster, →"Iteration Duration RT Timed-Loop":i64)
